vi "VP_RT_MultiTraj.vi"() -> ()   [LabVIEW 2015]
uses:
  Local or Remote.ctl
  State Enum.ctl
  Command Enum.ctl
  Controller Type.ctl
  EPICS Command Control.ctl
  <vilib>/Platform/TimedLoop/XDataNode/timing_clust.ctl
  <vilib>/Platform/TimedLoop/XDataNode/nitl_modes.ctl
  <vilib>/Platform/TimedLoop/XDataNode/wakeup.ctl
  Data Write Control.ctl
  <vilib>/FPGAPlugInAG/cRIO-9039/niLvFpga_Open_cRIO-9039.vi
  <vilib>/rvi/interface/common/dynamic/niFpgaDynamicAddResources.vi
  <vilib>/Utility/error.llb/Error Cluster From Error Code.vi
  <vilib>/rvi/errors/niLvFpgaAdjustHostInterfaceError.vi
  <vilib>/rvi/interface/common/niFpgaWaitOnOcc.vi
  <vilib>/FPGAPlugInAG/Dynamic/niLvFpga_Reset_Dynamic.vi
  <vilib>/FPGAPlugInAG/Dynamic/niLvFpga_Abort_Dynamic.vi
  <vilib>/FPGAPlugInAG/Dynamic/niLvFpga_Close_Dynamic.vi
  <vilib>/Platform/TimedLoop/XDataNode/XDataNode.xnode
  <vilib>/rvi/interface/nirviOpenFPGA/nirviOpenFPGA.xnode
  FPGA Bitfiles/VP_NanoPositioner_FPGA_MultiTraj.lvbitx
  <vilib>/rvi/interface/nirviReadWriteControl/nirviReadWriteControl.xnode
  <vilib>/rvi/interface/nirviMethod/nirviMethod.xnode
  <vilib>/rvi/interface/nirviCloseFPGA/nirviCloseFPGA.xnode
  <vilib>/Platform/TimedLoop/XDataNode/XDNodeRunTimeDep.lvlib
  <vilib>/rvi/errors/niLvFpgaMergeErrorWithErrorCode.vi
  NiFpgaLv.dll
  <vilib>/rvi/interface/Simulation/niFpgaSimulationCallBeginRW.vi
  <vilib>/rvi/Analysis/host/Public/NI_FpgaMspHost.lvlib
  <vilib>/FPGAPlugInAG/Dynamic/niLvFpga_StopFifo_Dynamic.vi
  <vilib>/FPGAPlugInAG/Dynamic/niLvFpga_ReadFifo_Dynamic.vi
  <vilib>/NI_Real-Time Target Support.lvlib
  <vilib>/FPGAPlugInAG/Dynamic/niLvFpga_ConfigureFifo_Dynamic.vi
  <vilib>/FPGAPlugInAG/Dynamic/niLvFpga_StartFifo_Dynamic.vi
panel:
  out "Kzz Output, Kzz*ez (V)":fxp<+/-,58,25>
  out "Kyy Output, Kyy*ey (V)":fxp<+/-,58,25>
  out "Kxx Output, Kxx*ex (V)":fxp<+/-,58,25>
  out "Controller Output Upper Limit Readback":fxp<+/-,20,5>
  out "Controller Output Lower Limit Readback":fxp<+/-,20,5>
  out "X-Stage Input In Range?":bool=TRUE
  out "Y-Stage Input In Range?":bool=TRUE
  out "Z-Stage Input In Range?":bool=TRUE
  in  "Tab Control":T1(tab)
  in  "Controller Type":T2
  in  "X Ramp Start (nm)":fxp<+/-,32,16>=-500.0
  in  "X Ramp End (nm)":fxp<+/-,32,16>=500.0
  in  "Y Ramp Start (nm)":fxp<+/-,32,16>=500.0
  in  "Y Ramp End (nm)":fxp<+/-,32,16>=-500.0
  in  "Y Step Size (nm)":fxp<+/-,32,16>=50.0
  in  "X Step Size (nm)":fxp<+/-,32,16>=50.0
  in  "System Loop Type":enum16{"Open Loop", "Closed Loop"}(ring)
  in  "DT Frequency (Hz)":dbl=1000.0 format="%#_6p"
  in  "DT duty cycle (%)":dbl=88.0 min=0.0 max=100.0 step=1.0
  in  "Max radius":fxp<+/-,32,16>
  in  "Spiral Step Size":fxp<+/-,32,16>
  in  "Scan Geometry":T3(ring)
  in  "Inner Scan axis":enum16{"X", "Y"}(ring)
  in  "Rotation Direction":enum16{"Clockwise", "Anti-clockwise"}(ring)
  in  "Radial direction":enum16{"Outward", "Inward"}(ring)
  out "Trajectory Completed":bool
  out "XY Ref":cluster{dbl[], dbl[]}[](graph)
  out "Elements Available in FIFO":u32(graph)
  out "Elements Remaining in FIFO":u32(graph)
  out "Reference and Actual positions":cluster{"t0":dbl, dbl, dbl[][]}(graph)
  in  "Timeout FPGA FIFO1":i32=40000000
  out "FIFO Timed Out":bool
  out "Stop Run":bool
  in  "Datalog Cases":T4(ring)=enum."Data Log 16"
  out "FIFO Timed Out?":bool
  out "Data Read Rate (Hz)":dbl=25000.000000000004
  out "Elements Remaining":u32
  in  "FIFO Timeout (ms)":i32=2500
  out "Actual Depth":u32=131068416
  in  "Requested Depth":u32=131068000
  in  "Fly scan loop dt":i64=250
  in  "Start Scan Loop dt":i64=50
  out "Queue is empty":bool=TRUE
  out "2iddVELO:VP:X_End_nm":dbl=2000.0
  out "2iddVELO:VP:X_Start_nm":dbl=-2000.0
  out "EPICS Execute Command":bool
  out "2iddVELO:VP:Y_Start_nm":dbl=2000.0
  out "2iddVELO:VP:Y_End_nm":dbl=-2000.0
  out "2iddVELO:VP:Y_Step_Size_nm":dbl=50.0
  out "2iddVELO:VP:X_Step_Size_nm":dbl=50.0
  out "2iddVELO:VP:Trigger_Freq_Hz":dbl=1000.0
  out "2iddVELO:VP:Trig_DutyCycle_Per":dbl=99.0
  out "Remote Mode":bool
  out "EPICS Controller Type":T2
  out "EPICS cRIO Command":T5
  out "EPICS Scan Trajectory":T3(ring)
  out "2iddVELO:VP:Max_Radius":dbl
  out "2iddVELO:VP:Spiral_Step":dbl
  out "Iteration Duration RT Timed-Loop":i64=128
  out "# of Hor Lines":fxp<+/-,64,34>=181.0 format="%.22g"
  out "# of Points per Line":fxp<+/-,33,17>=180.0
  out "# Total Trigger Points":fxp<+/-,64,34>=32580.0
  out "sec per line":dbl=0.06
  out "line per sec (Hz)":dbl=16.666666666666668
  out "Total Scan Time (sec)":dbl=10.86
  in  "Controller Time Period (uSec)":u32=40
  in  "Controller Output Time Period (uSec)":u32=40
  in  "XY Reference Time Period (uSec)":u32=40
  in  "Plant Output Time Period (uSec)":u32=40
  in  "Datalog Time Period (uSec)":u32=40
  in  "Trigger Generation Time Period (uSec)":u32=40
  in  "Z Reference Time Period (uSec)":u32=40
  in  "Stop System (Careful!!)":bool
  in  "Reset All":bool
  in  "Base name":string="base_name"
  out "Mod6/DIO3":bool
  out "Mod5/DIO3":bool
  out "Mod4/DIO3":bool
  in  "Sample Z Stage Resolution (nm)":fxp<+,33,3>=0.5
  in  "Sample Y Stage Resolution (nm)":fxp<+,33,3>=0.5
  in  "Sample X Stage Resolution (nm)":fxp<+,33,3>=0.5
  in  "Optics Z Stage Resolution (nm)":fxp<+,33,3>=0.5
  in  "Optics Y Stage Resolution (nm)":fxp<+,33,3>=0.5
  in  "Optics X Stage Resolution (nm)":fxp<+,33,3>=0.5
  in  "Sample Z Reset":bool
  in  "Sample Y Reset":bool
  in  "Sample X Reset":bool
  out "Mod6/DIO2":bool
  out "Mod6/DIO1":bool
  out "Mod6/DIO0":bool=TRUE
  out "Mod5/DIO2":bool
  out "Mod5/DIO1":bool=TRUE
  out "Mod5/DIO0":bool
  out "Mod4/DIO2":bool=TRUE
  out "Mod4/DIO1":bool
  out "Mod4/DIO0":bool=TRUE
  in  "Optics Z Reset":bool
  in  "Optics Y Reset":bool
  in  "Optics X Reset":bool
  in  "Detector Trigger Lower Limit (V)":fxp<+/-,20,5>
  in  "Detector Trigger Upper Limit (V)":fxp<+/-,20,5>=5.0
  out "Detector Trigger In Range?":bool=TRUE
  in  "DT Reference Amplitude (V)":fxp<+/-,40,17>=5.0
  in  "DT Reference DC Offset (V)":fxp<+/-,16,16>
  out "DT Frequency (periods/tick)":fxp<+,32,0>=7.500010542571545e-05
  out "DT Phase Offset (periods)":fxp<+,32,0>
  in  "DT Reset":bool
  out "DT Duty Cycle (periods)":fxp<+,32,0>=0.8799999998882413
  in  "DT phase offset (deg)":dbl format="%#.6g"
  out "Trigger Frequency (Hz)":dbl
  out "Trigger Duty Cycle (%)":dbl
  in  "Scaling mV to V":fxp<+,33,10>=0.001000046730041504
  out "Heartbeat":bool=TRUE
  in  "System command":T6
  in  "Execute":bool
  out "Last Command Executed":T6
  in  "Optics and or Sample Stage":T7(ring)
  in  "Local_Lock":bool
  out "Local or EPICS":T8
  out "Output filename":string
  out "Output path":path
  out "FPGA state":T9(ring)
  in  "cRIO data dir":string="/home/lvuser/natinst/data"
  out "RT Main Loop State":T10
  out "cRIO path":path
  out "Iteration Duration":i64
  out "Controller loop iterations":i32
  out "Z Reference Loop iterations":i32
  out "XY Reference Loop iterations":i32
  out "FIFO loop iterations":i32
  out "Trigger Generation Loop iterations":i32
  out "Module output loop iterations":i32
  out "Plant output loop iterations":i32
  in  "Data Save Trigger Source":enum16{"Detector", "Trajectory"}(ring)
  out "EPICS rotation direction":enum16{"Clockwise", "Anti-clockwise"}(ring)
  out "EPICS radial direction":enum16{"Outward", "Inward"}(ring)
  out "EPICS Inner axis":enum16{"X", "Y"}(ring)
  out "Optics Z Stage Displacement (nm)":fxp<+/-,32,16>
  out "Optics Y Stage Displacement (nm)":fxp<+/-,32,16>
  out "Optics X Stage Displacement (nm)":fxp<+/-,32,16>=-1.0
  in  "Scan type":enum16{"Fly", "Step"}(ring)
  out "EPICS Scan Type":enum16{"Fly", "Step"}(ring)
  out "Counter Loop iterations":i32
  out "Outer Loop iterations":i32
  out "Scan Type and Geometry":T11(ring)
  out "Position Number":u32
  in  "Data Save Flag":enum16{"Skip Data", "Save Data"}(ring)=enum."Save Data"
  in  "Z-Stage Scaling Direction":fxp<+/-,3,3>=-1.0
  in  "Y-Stage Scaling Direction":fxp<+/-,3,3>=-1.0
  in  "Z-Stage nm to V Scaling":fxp<+/-,32,12>=0.0005397796630859375
  in  "Y-Stage nm to V Scaling":fxp<+/-,32,12>=0.0014200210571289062
  in  "X-Stage Scaling Direction":fxp<+/-,3,3>=-1.0
  in  "X-Stage nm to V Scaling":fxp<+/-,32,12>=0.0005359649658203125
  in  "Controller Output Lower Limit":fxp<+/-,20,5>=-5.0
  in  "Controller Output Upper Limit":fxp<+/-,20,5>=5.0
  in  "FPGA Wait Timer (ms)":u16=5
  in  "Pre-Scan pause (ms)":u32=250
  in  "Readback Loop time between iterations (ms)":u32=10
  in  "Z Reference DC Offset (nm)":fxp<+/-,15,15>
  in  "Y Reference DC Offset (nm)":fxp<+/-,16,16>
  in  "X Reference DC Offset (nm)":fxp<+/-,16,16>
  in  "Z Reference Amplitude (nm)":fxp<+/-,40,17>
  in  "Y Reference Amplitude (nm)":fxp<+/-,40,17>=100.0
  in  "X Reference Amplitude (nm)":fxp<+/-,40,17>=100.0
  out "Trajectory frequency (periods/tick)":fxp<+,32,0>=1.25030055642128e-07 format="%#.5e"
  in  "Trajectory frequency (Hz)":dbl=25000.0 format="%#_6p"
  out "actual Traj frequency (Hz)":dbl format="%#_6p"
  out "Measured Datalog Time Period (Ticks)":u32=1600
  out "Measured Datalog Loop Rate (us)":dbl=3.9999999999999996e-05
  out "Measured Datalog Loop Rate (kHz)":dbl=25.000000000000004
  out "Measured Counter Loop Rate (us)":dbl
  out "Measured Counter Loop Rate (MHz)":dbl=inf
  out "Measured XY Reference Loop Rate (us)":dbl=3.9999999999999996e-05
  out "Measured XY Reference Loop Rate (kHz)":dbl=25.000000000000004
  out "Measured XY Reference Time Period (Ticks)":u32=1600
  out "Measured Controller Loop Rate (kHz)":dbl=25.000000000000004
  out "Measured Controller Output Loop Rate (us)":dbl=3.9999999999999996e-05
  out "Measured Controller Output Loop Rate (kHz)":dbl=25.000000000000004
  out "Measured Plant Output Loop Rate (us)":dbl=3.9999999999999996e-05
  out "Measured Plant Output Loop Rate (kHz)":dbl=25.000000000000004
  out "Measured Controller Loop Rate (us)":dbl=3.9999999999999996e-05
  out "Measured Controller Time Period (Ticks)":u32=1600
  out "Data Read Period (sec)":dbl=3.9999999999999996e-05
  out "Measured Controller Output Time Period (Ticks)":u32=1600
  out "Measured Plant Output Time Period (Ticks)":u32=1600
  out "Measured Counter Time Period (Ticks)":u32
  out "Measured Trigger Gen Time Period (Ticks)":u32=1600
  out "Measured Z Reference Time Period (Ticks)":u32=1600
  out "Measured Z Reference Loop Rate (us)":dbl=3.9999999999999996e-05
  out "Measured Z Reference Loop Rate (kHz)":dbl=25.000000000000004
  out "Number of Data Strings":i32=5
  out "Data":fxp<+/-,40,32>[](array[numeric])
  out "Measured Trigger Gen Loop Rate (us)":dbl=3.9999999999999996e-05
  out "Measured Trigger Gen Loop Rate (kHz)":dbl=25.000000000000004
  in  "file path soscoeff_xx1 Hinf":path=path "/home/lvuser/natinst/controllers/Kxx_1_Gxx_matched_dow_16ord_mVpnm_cd8a3_AvTio9_X5nm_500pm_all_40us_soscof_xx1.mat"
  in  "file path sos gain SF Controller_xx1 Hinf":path=path "/home/lvuser/natinst/controllers/Kxx_1_Gxx_matched_dow_16ord_mVpnm_cd8a3_AvTio9_X5nm_500pm_all_40us_soscof_xx2.mat"
  in  "file path soscoeff_yy1 Hinf":path=path "/home/lvuser/natinst/controllers/Kyy_trial_1_Gyy_matched_dow_8ord_mVpnm_cd8a3_AvTio9_Y5nm_500pm_all_40us_soscof_yy1.mat"
  in  "file path sos gain SF Controller_yy1 Hinf":path=path "/home/lvuser/natinst/controllers/Kyy_trial_1_Gyy_matched_dow_8ord_mVpnm_cd8a3_AvTio9_Y5nm_500pm_all_40us_soscof_yy2.mat"
  in  "file path soscoeff_zz1 Hinf":path=path "/home/lvuser/natinst/controllers/Kzz_1_Gzz_matched_dow_29ord_mVpnm_cd8a3_AvTio9_Z5nm_500pm_all_40us_soscof_zz1.mat"
  in  "file path sos gain SF Controller_zz1 Hinf":path=path "/home/lvuser/natinst/controllers/Kzz_1_Gzz_matched_dow_29ord_mVpnm_cd8a3_AvTio9_Z5nm_500pm_all_40us_soscof_zz2.mat"
  in  "file path soscoeff_xx1 PID":path=path "/home/lvuser/natinst/controllers/Kxx_pid_2_Gxx_tustin_2ord_mVpnm_cd8a3_soscof_xx1.mat"
  in  "file path sos gain SF Controller_xx1 PID":path=path "/home/lvuser/natinst/controllers/Kxx_pid_2_Gxx_tustin_2ord_mVpnm_cd8a3_soscof_xx2.mat"
  in  "file path soscoeff_yy1 PID":path=path "/home/lvuser/natinst/controllers/Kyy_pid_4_Gyy_tustin_2ord_mVpnm_cd8a3_soscof_yy1.mat"
  in  "file path sos gain SF Controller_yy1 PID":path=path "/home/lvuser/natinst/controllers/Kyy_pid_4_Gyy_tustin_2ord_mVpnm_cd8a3_soscof_yy2.mat"
  in  "file path soscoeff_zz1 PID":path=path "/home/lvuser/natinst/controllers/Kzz_pid_2_Gzz_tustin_2ord_mVpnm_cd8a3_soscof_zz1.mat"
  in  "file path sos gain SF Controller_zz1 PID":path=path "/home/lvuser/natinst/controllers/Kzz_pid_2_Gzz_tustin_2ord_mVpnm_cd8a3_soscof_zz2.mat"
  out "-a01(2) xx1c":fxp<+/-,64,9>[](array[numeric])=[0.637785025840232, 0.9924182654286198, 1.8461027816316544, 0.8635404845716299, 1.0670555456779864, 1.6350703383821101, 1.6323955588345012, 1.1102241390539636, 0.0, 0.0, 0.0, 0.0, 0.0, 0.0, 0.0, 0.0, 0.0, 0.0, 0.0, 0.0]
  out "-a02(2) xx1c":fxp<+/-,64,9>[](array[numeric])=[-0.999855815746439, -0.9676991072632725, -0.9642268720534838, -0.9446498323360957, -0.9442808087139987, -0.7547983908829242, -0.6690016013017409, -0.11027986125857198, 0.0, 0.0, 0.0, 0.0, 0.0, 0.0, 0.0, 0.0, 0.0, 0.0, 0.0, 0.0]
  out "b01(2) xx1c":fxp<+/-,64,9>[](array[numeric])=[-0.6378105164532328, -1.0062332697665268, -1.8762916543815855, -0.8616288879491845, -1.0856571140792324, -1.6862585929720944, -1.743591709663851, -0.6129835805090948, 0.0, 0.0, 0.0, 0.0, 0.0, 0.0, 0.0, 0.0, 0.0, 0.0, 0.0, 0.0]
  out "b02(2) xx1c":fxp<+/-,64,9>[](array[numeric])=[0.9999102047610771, 0.9971375605901365, 0.9926840301018772, 0.9509648854364836, 0.9563369558920378, 0.7818900462139817, 0.7642575436257291, 3.0531133177191805e-16, 0.0, 0.0, 0.0, 0.0, 0.0, 0.0, 0.0, 0.0, 0.0, 0.0, 0.0, 0.0]
  out "sos gain SF Controller xx1c":fxp<+/-,42,9>=-0.1625035791657865
  out "-a01(2) yy1c":fxp<+/-,64,9>[](array[numeric])=[1.8740229377643998, 1.3096977339382483, 1.7453886241944765, 0.2668895009727739, 0.0, 0.0, 0.0, 0.0, 0.0, 0.0, 0.0, 0.0, 0.0, 0.0, 0.0, 0.0, 0.0, 0.0, 0.0, 0.0]
  out "-a02(2) yy1c":fxp<+/-,64,9>[](array[numeric])=[-0.9732703278433918, -0.5194903821190732, -0.7453924481836136, -2.7755575615628914e-17, 0.0, 0.0, 0.0, 0.0, 0.0, 0.0, 0.0, 0.0, 0.0, 0.0, 0.0, 0.0, 0.0, 0.0, 0.0, 0.0]
  out "b01(2) yy1c":fxp<+/-,64,9>[](array[numeric])=[-1.8979173162254057, -1.8463149313261074, -1.7151162246453355, -0.006444279582847878, 0.0, 0.0, 0.0, 0.0, 0.0, 0.0, 0.0, 0.0, 0.0, 0.0, 0.0, 0.0, 0.0, 0.0, 0.0, 0.0]
  out "b02(2) yy1c":fxp<+/-,64,9>[](array[numeric])=[0.9969084979865663, 0.9421233904433339, 0.7362048104846675, 0.0, 0.0, 0.0, 0.0, 0.0, 0.0, 0.0, 0.0, 0.0, 0.0, 0.0, 0.0, 0.0, 0.0, 0.0, 0.0, 0.0]
  out "sos gain SF Controller yy1c":fxp<+/-,42,9>=-1.480983349494636
  out "-a01(2) zz1c":fxp<+/-,64,9>[](array[numeric])=[0.6242394224317618, 1.8967038692417004, 0.6659160318030806, 1.7792660019034106, 1.6870099721477447, 0.6417945190222861, 1.4838029149808185, 1.8456549628851837, 1.2189509782386598, 0.9933314517253298, 1.0158915520299678, 0.8863484387433826, 0.026837806879254994, 1.8269783715122585, 0.22448441435364225, 0.0, 0.0, 0.0, 0.0, 0.0]
  out "-a02(2) zz1c":fxp<+/-,64,9>[](array[numeric])=[-0.9983298461163967, -0.9972287452752734, -0.995744457243837, -0.9947210838396919, -0.9925914602095722, -0.9920974045271405, -0.9881915357970101, -0.9800069383591395, -0.9760641145386646, -0.9508624135515895, -0.9242774595356998, -0.655945641403593, -0.008661844724279444, -0.8269827070369743, 0.0, 0.0, 0.0, 0.0, 0.0, 0.0]
  out "b01(2) zz1c":fxp<+/-,64,9>[](array[numeric])=[-0.6245671059510156, -1.897930093390194, -0.6670970070931089, -1.7670265604573054, -1.6833314913922348, -0.6327437892303018, -1.5025901530730128, -1.8636454269915796, -1.1210694827766767, -0.9982206064398196, -1.0326369335418408, -1.1342635673267367, -1.6852506306166828, -0.9843740162364313, -1.7208456881689926e-15, 0.0, 0.0, 0.0, 0.0, 0.0]
  out "b02(2) zz1c":fxp<+/-,64,9>[](array[numeric])=[0.9973135069419645, 0.9951302056171929, 0.9993435624612031, 0.9919371251860779, 0.994931751453586, 0.9881092761723503, 0.9884874399279107, 0.9977145546300196, 0.9725302934743221, 0.9855561672767964, 0.9893454712398023, 0.846212786518208, 0.7855598927779743, 0.0978075435519738, 0.0, 0.0, 0.0, 0.0, 0.0, 0.0]
  out "sos gain SF Controller zz1c":fxp<+/-,42,9>=-0.1988595259608701
  out "FPGA error monitor":errorcluster
  out "FPGA end run error":errorcluster
  out "Timed Loop (end error)":errorcluster
  out "Main Loop error":errorcluster
  out "Main Loop Iterations":i32
  out "RT error":errorcluster
  out "Command Loop Error":errorcluster
  out "Readback error":errorcluster
  out "FPGA wait error":errorcluster
  out "Coeff file import error":errorcluster
  out "Readback loop Iterations":i32
  out "Command Loop Iterations":i32
  out "Heartbeat Loop Iterations":i32
  out "EPICS command error":errorcluster
  out "FPGA Run Loop error":errorcluster
  out "File Writer loop error":errorcluster
  out "File writer loop iterations":i32
  out "Reduced Array of States":T10[](array[typedef])
  out "2iddVELO:VP:Scan_Type":string
  out "2iddVELO:VP:Controller_Type":string
  out "2iddVELO:VP:cRIO_Command":string
  out "2iddVELO:VP:Scan_Trajectory":string
  out "2iddVELO:VP:Radial_Direction":string
  out "2iddVELO:VP:Rotation_Direction":string
  out "2iddVELO:VP:Inner_Scan_Axis":string
  out "2iddVELO:VP:X_Center":dbl
  out "2iddVELO:VP:Y_Center":dbl
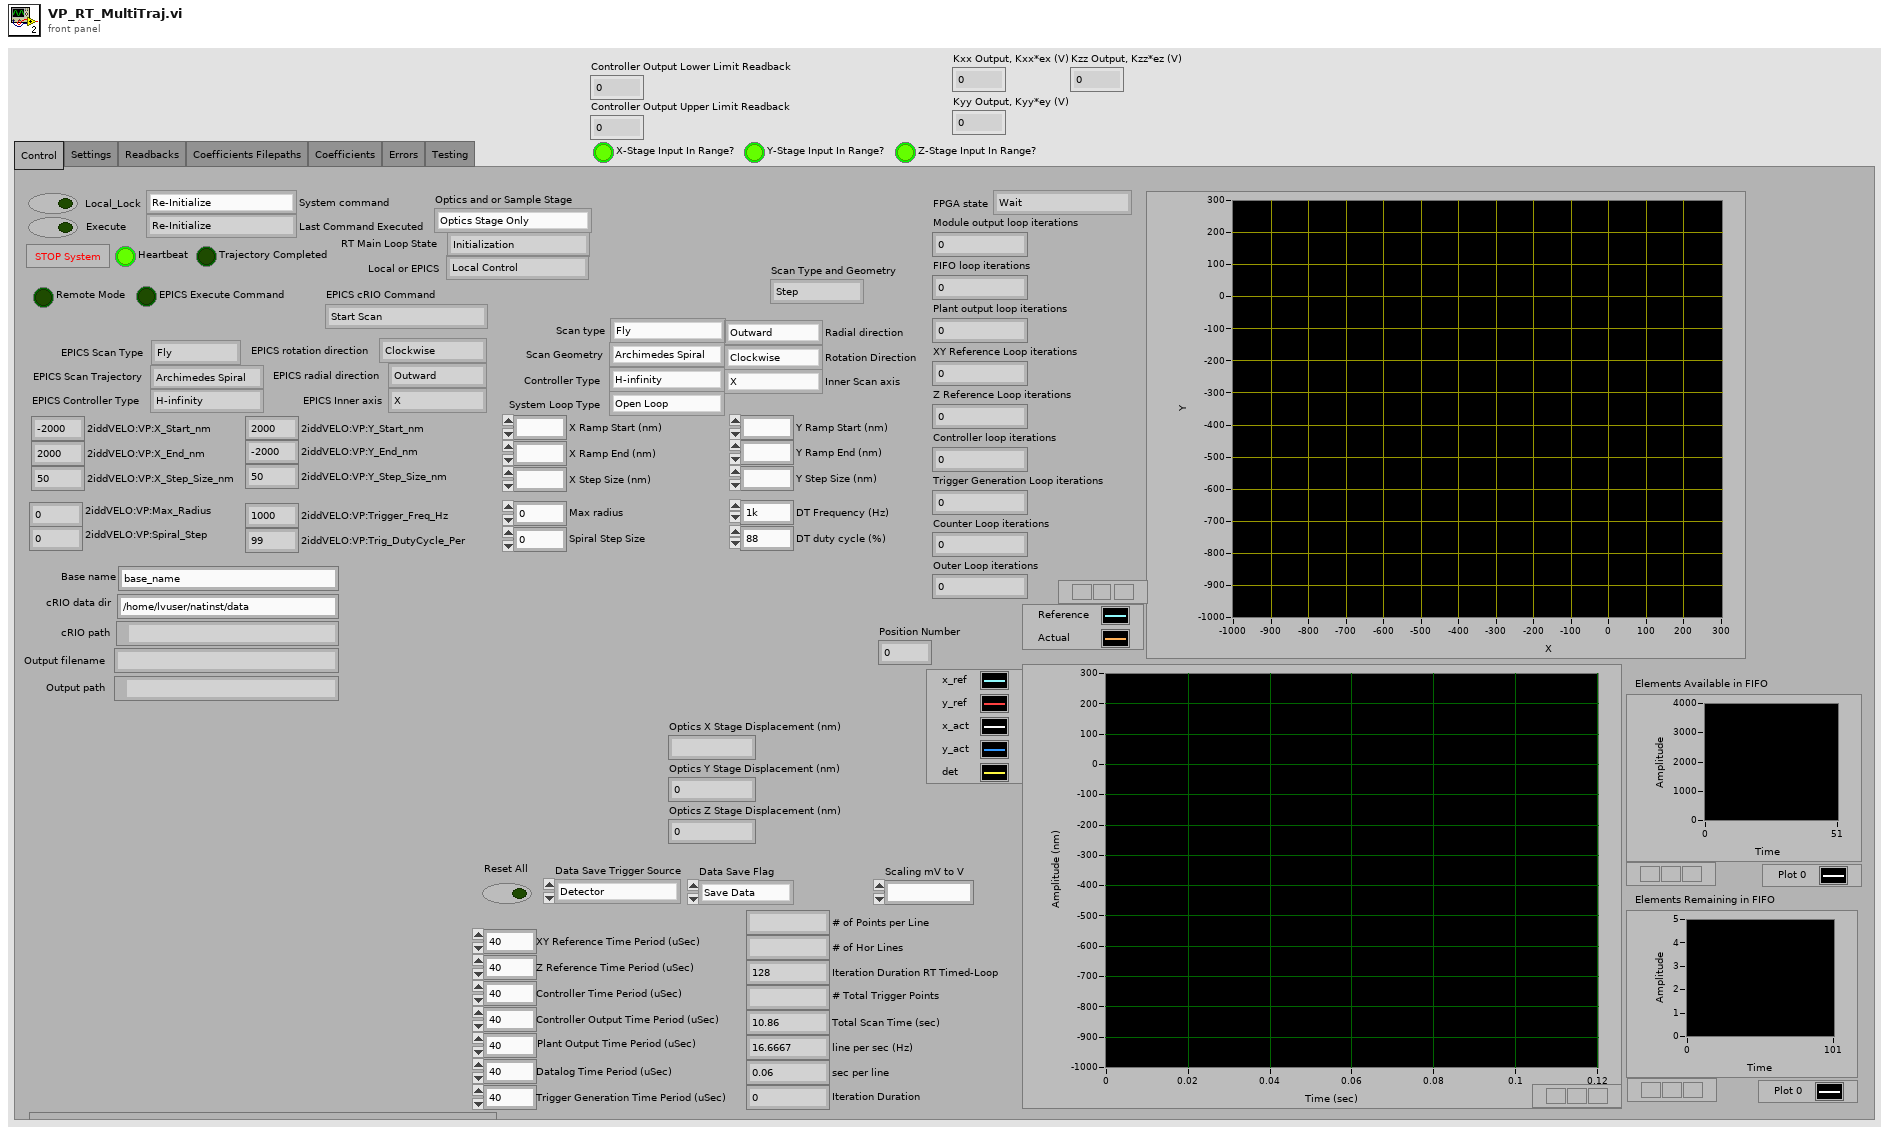
[diagram p1: front panel]
types:
  T1 = enum32{"Control", "Settings", "Readbacks", "Coefficients Filepaths", "Coefficients", "Errors", "Testing"}
  T2 = typedef "Controller Type.ctl" = enum16{"H-infinity", "PID"}
  T3 = enum16{"Archimedes Spiral", "Grid Spiral", "Snake"}
  T4 = enum16{"Data Log 1", "Data Log 2", "Data Log 3", "Data Log 4", "Data Log 5", "Data Log 6", "Data Log 7", "Data Log 8", "Data Log 9", "Data Log 10", "Data Log 11", "Data Log 12", "Data Log 13", "Data Log 14", "Data Log 15", "Data Log 16"}
  T5 = typedef "EPICS Command Control.ctl" = enum16{"Start Scan", "Stop Scan", "Reload Controller"}
  T6 = typedef "Command Enum.ctl" = enum16{"Re-Initialize ", "Update Scan Settings", "Scan", "Stop Scan", "Restart FPGA", "Stop System"}
  T7 = enum16{"Optics Stage Only", "Optics and Sample Stage"}
  T8 = typedef "Local or Remote.ctl" = enum16{"Local Control", "EPICS Control"}
  T9 = enum16{"Wait", "Start Run", "Run", "End Run", "Shutdown"}
  T10 = typedef "State Enum.ctl" = enum16{"Initialization", "Import Controller coeffs", "Update Controller Info", "Wait", "Update Reference Info", "Update Detector Trigger Info", "Update Datalog Info", "Check FPGA Status", "Initialize FIFO", "Pre-Scan", "Start Scan", "Step Scanning", "Fly Scanning", "End Scan", "Close File", "Restart FPGA", "Stop FPGA"}
  T11 = enum16{"Step", "Fly Arch Spiral", "Fly Snake", "Fly Grid Spiral"}
  T12 = typedef "XDNodeRunTimeDep.lvlib/timing_clust.ctl" = cluster{"Expected End [f-1]":u64, "Actual End [f-1]":u64, "Finished Late? [f-1]":bool, "Expected End [i-1]":u64, "Actual End [i-1]":u64, "Finished Late? [i-1]":bool, "Expected Start [i]":u64, "Actual Start [i]":u64, "Expected Start [f]":u64, "Actual Start [f]":u64, "Source Name":string, "Structure Name":string, "Period":i64, "Deadline":i64, "Offset":i64, "Start":i64, "Priority":i32, "Timeout":i32, "Mode":T13, "Wakeup Reason":T14, "Error":errorcluster, "Source Type":string, "Secondary Source Type":string, "Global End Time":u64, "Global Start Time":u64, "Frame Duration":u64, "Iteration Duration":u64, "Assigned CPU":i32, "I/O Scan Engine Mode":u32}
  T13 = typedef "XDNodeRunTimeDep.lvlib/nitl_modes.ctl" = enum32{"No Change", "Process missed periods, maintain original phase", "Discard missed periods, maintain original phase", "Process missed periods, ignore original phase", "Discard missed periods, ignore original phase"}
  T14 = typedef "XDNodeRunTimeDep.lvlib/wakeup.ctl" = enum32{"Normal", "Aborted", "Asynchronous wakeup", "Timing source error", "Timed loop error", "Timeout"}
  T15 = typedef "Data Write Control.ctl" = enum16{"Initialize", "Read", "Write", "Close"}
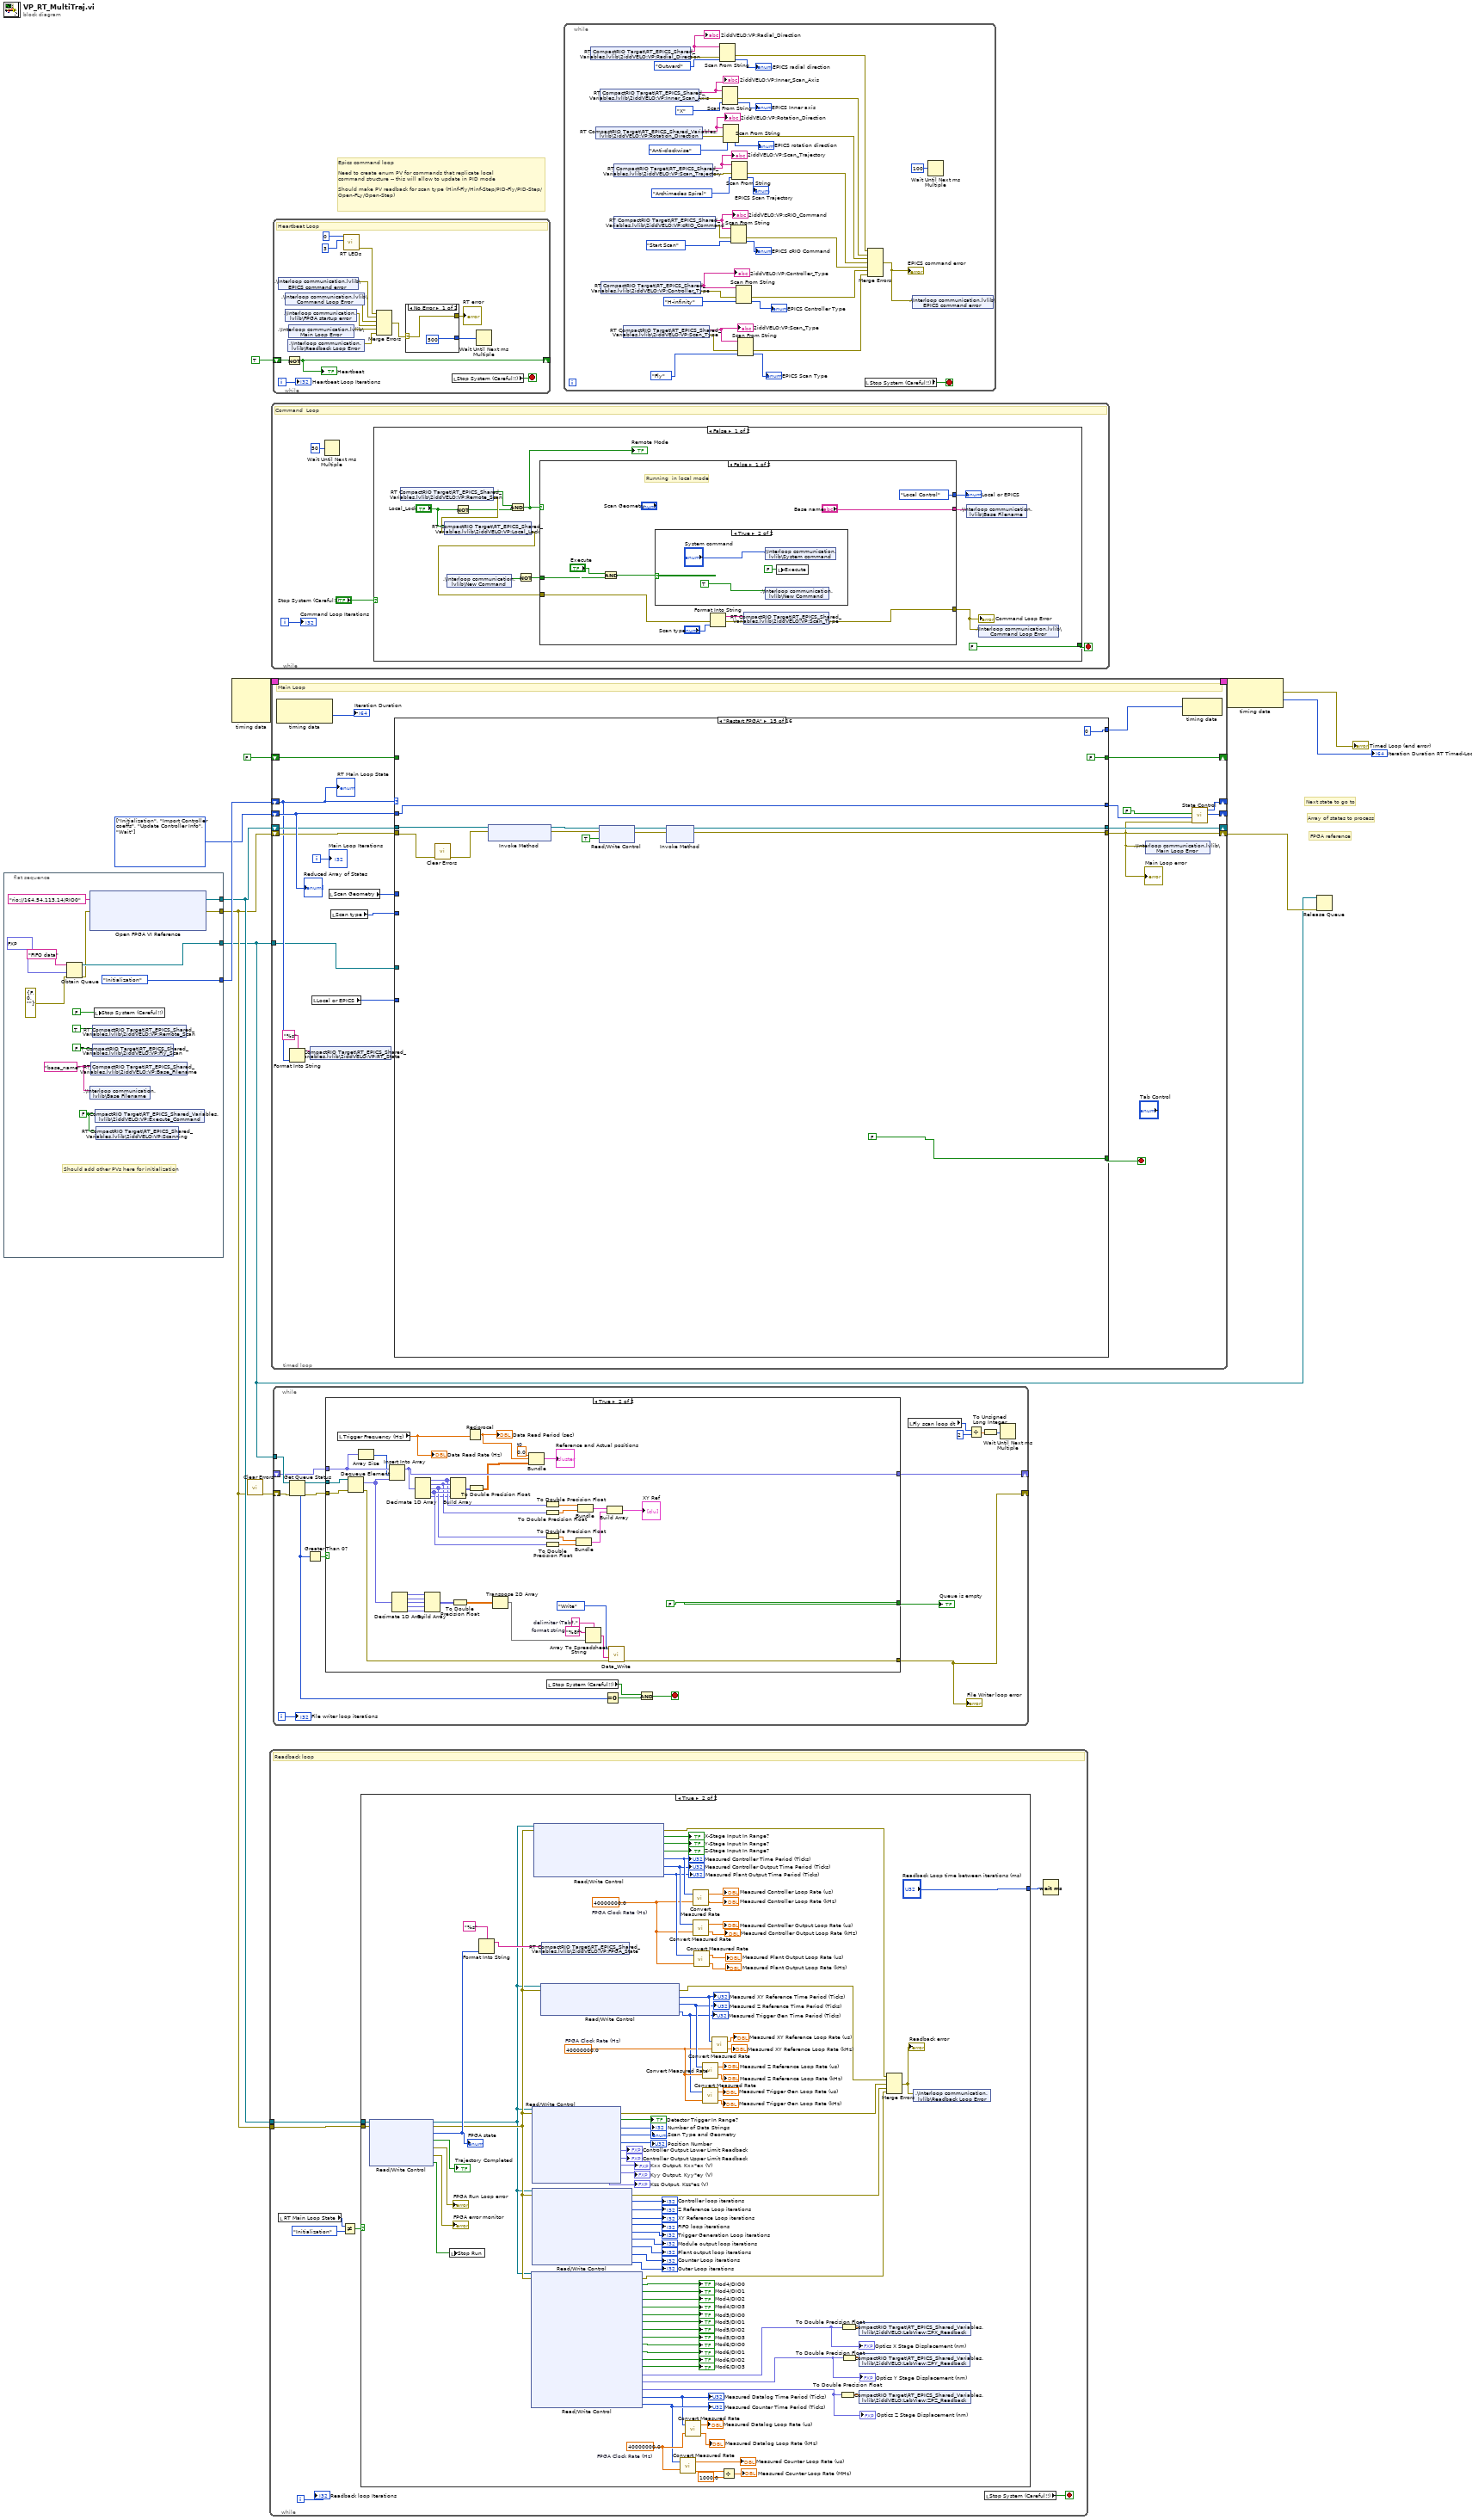
[diagram p0: block diagram]
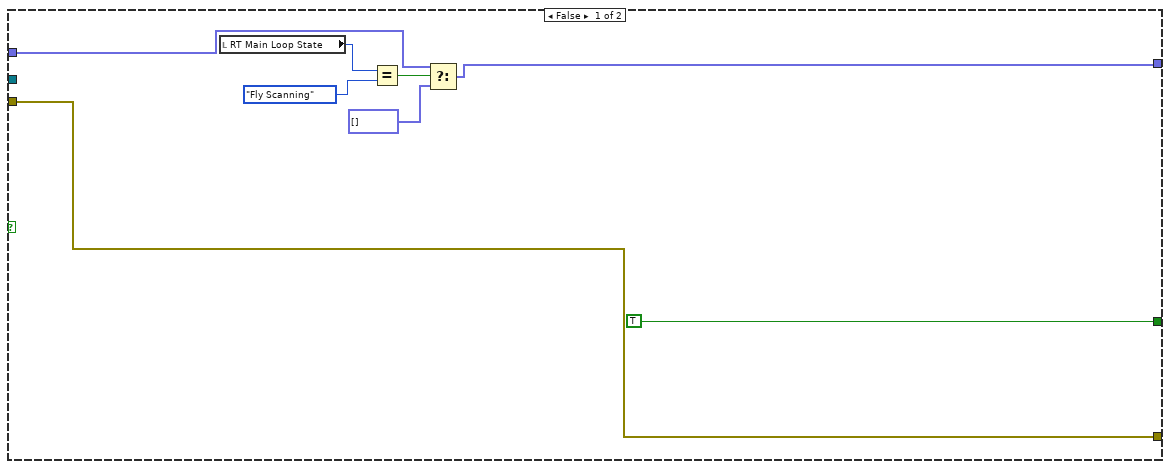
[diagram p2: hidden frame]
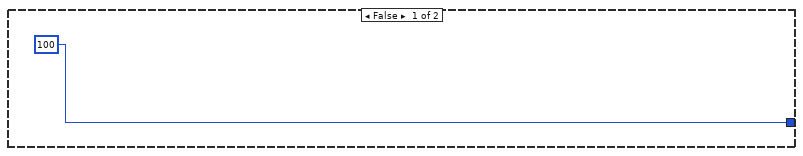
[diagram p3: hidden frame]
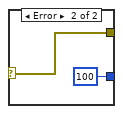
[diagram p4: hidden frame]
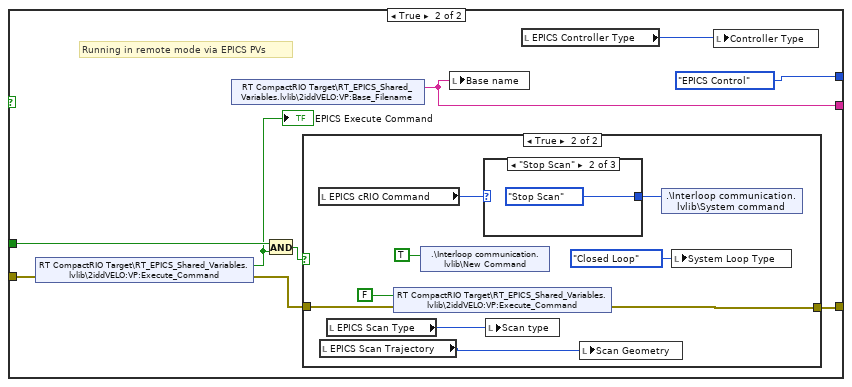
[diagram p6: hidden frame]
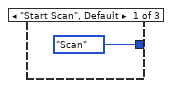
[diagram p8: hidden frame]
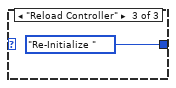
[diagram p9: hidden frame]
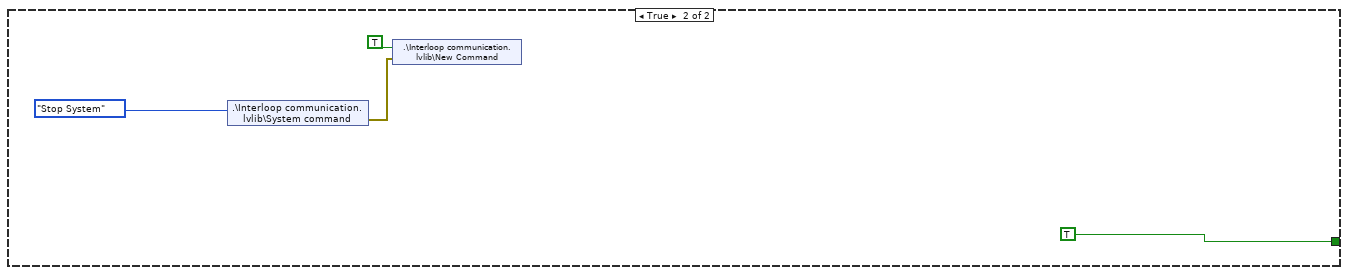
[diagram p10: hidden frame]
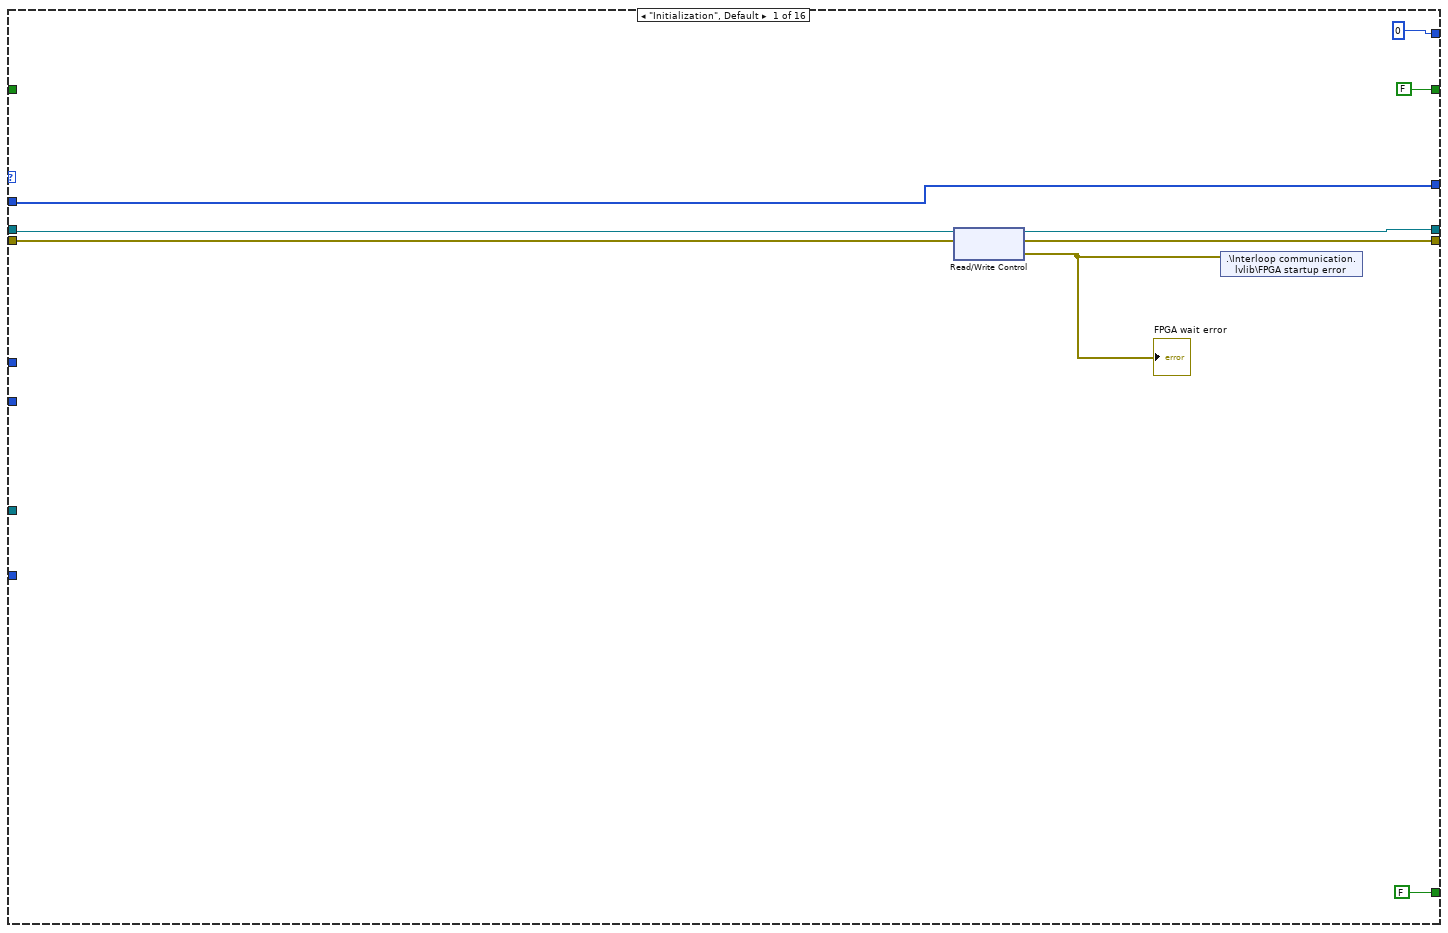
[diagram p11: hidden frame]
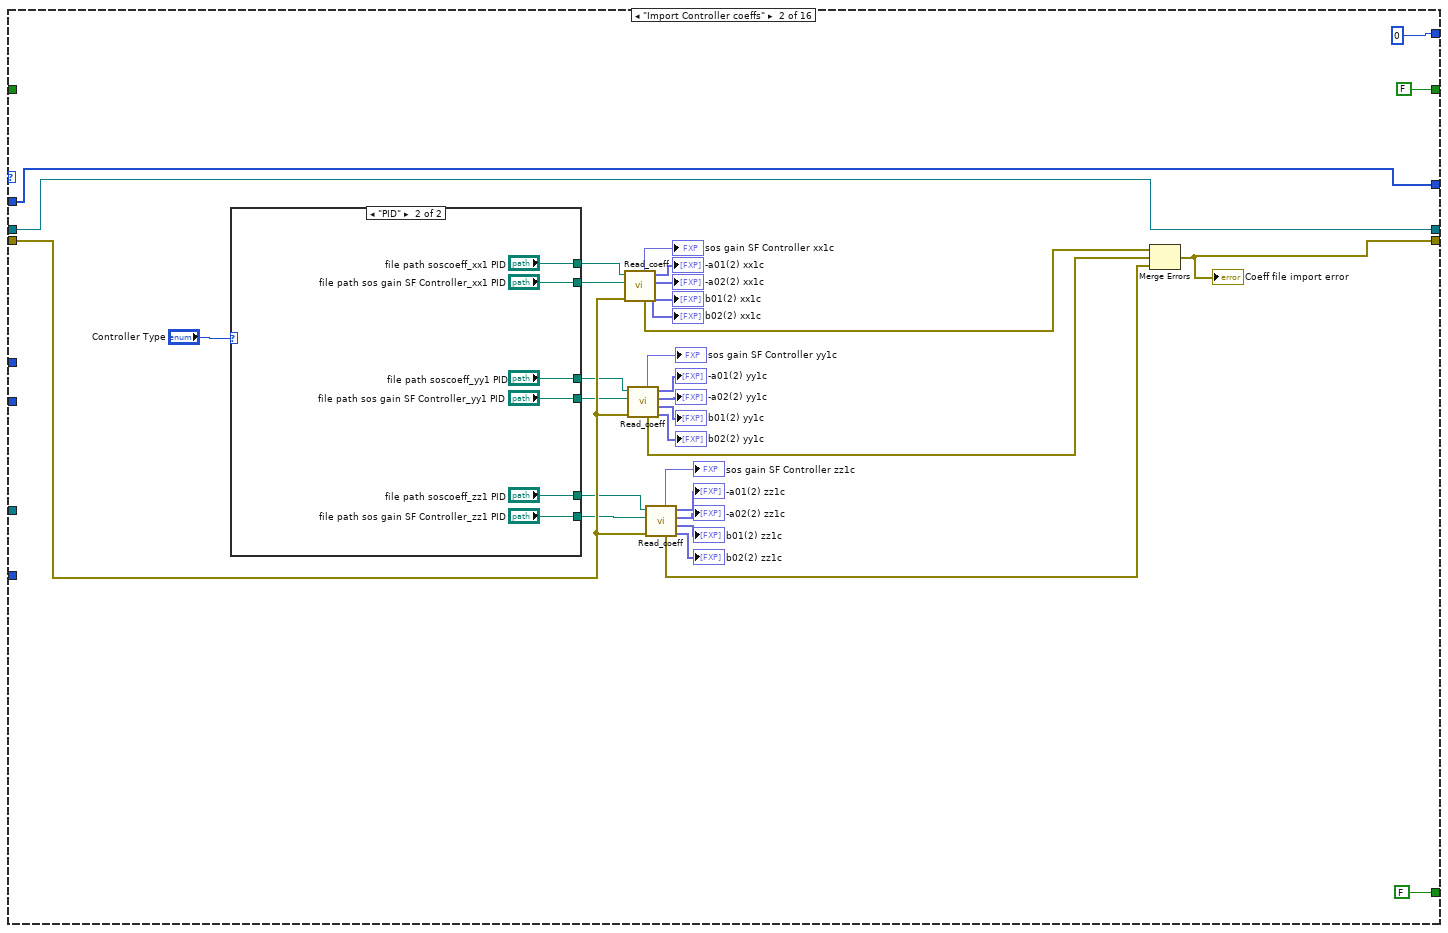
[diagram p12: hidden frame]
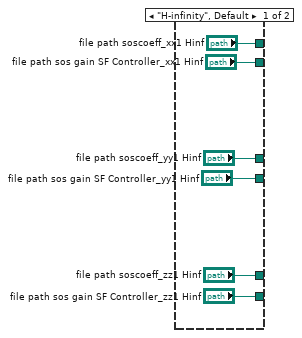
[diagram p13: hidden frame]
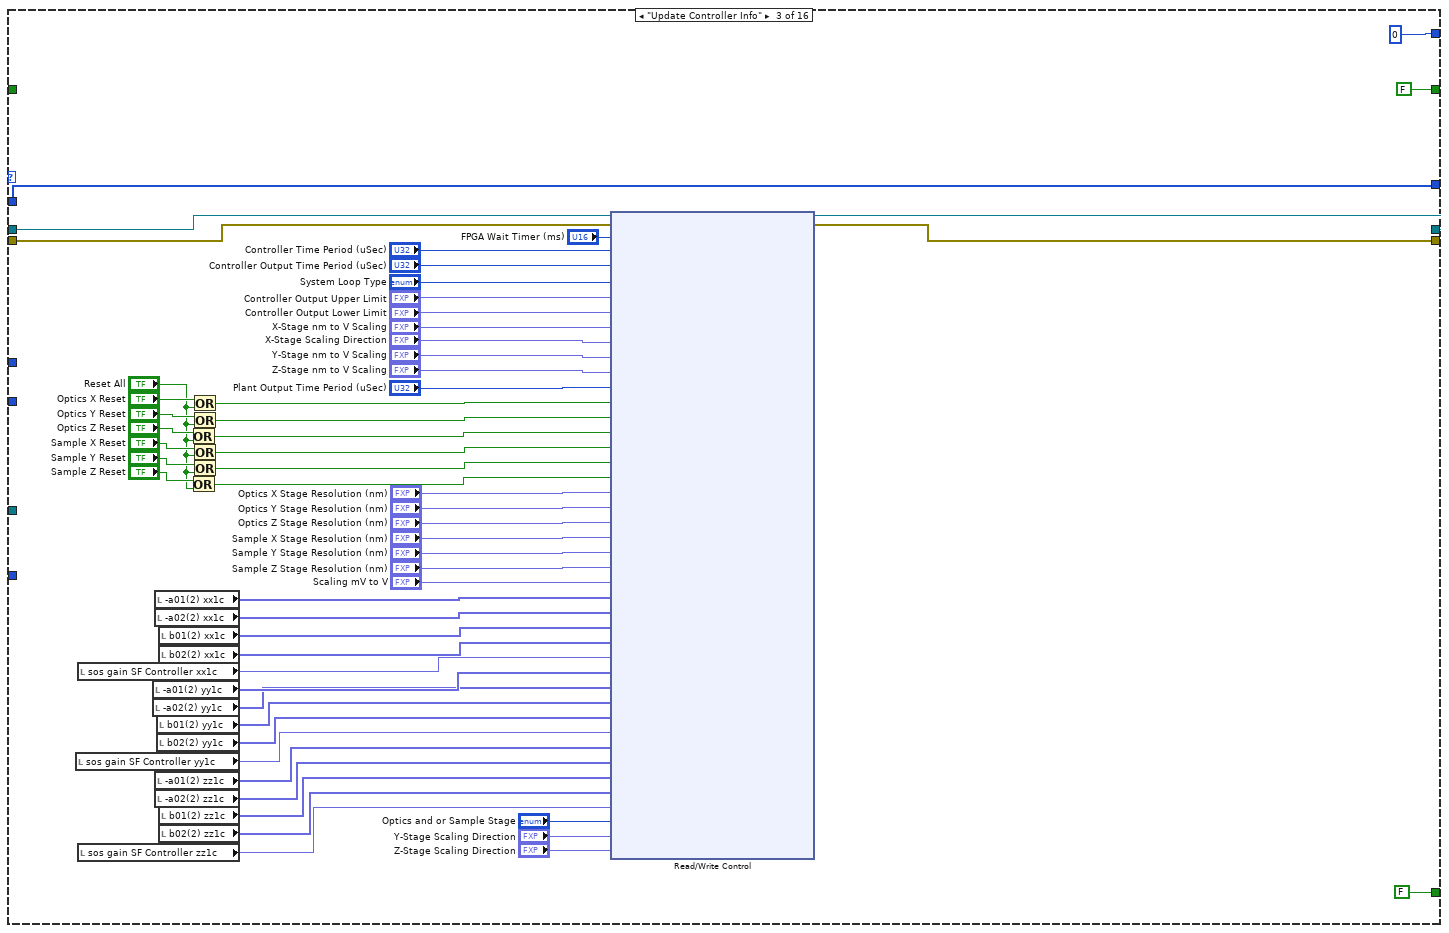
[diagram p14: hidden frame]
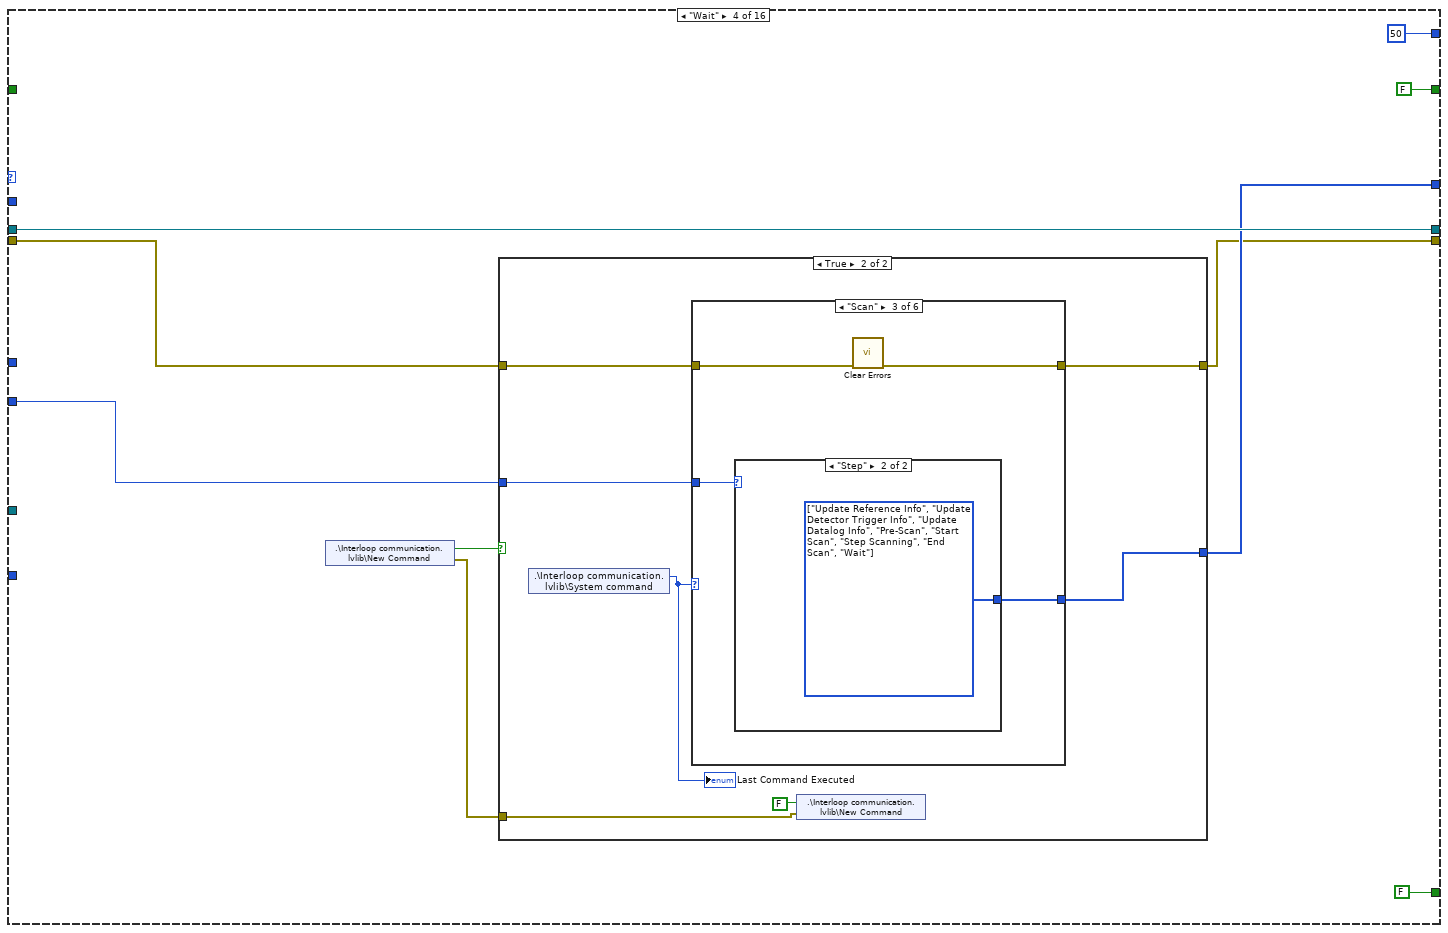
[diagram p15: hidden frame]
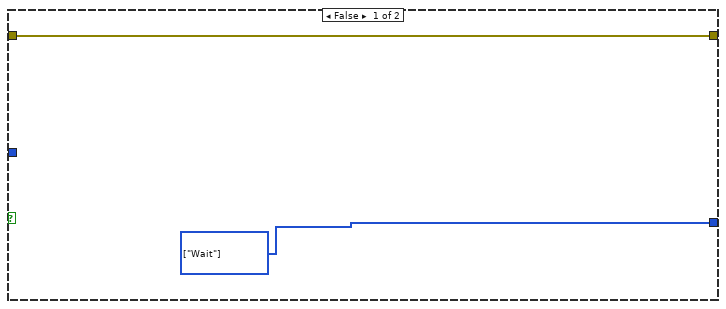
[diagram p16: hidden frame]
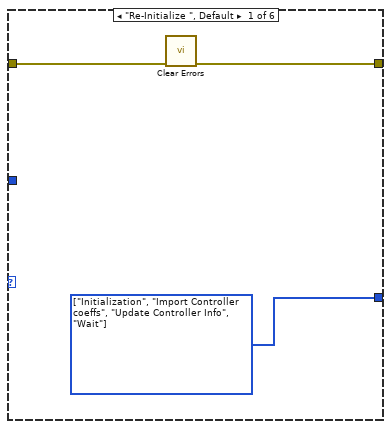
[diagram p17: hidden frame]
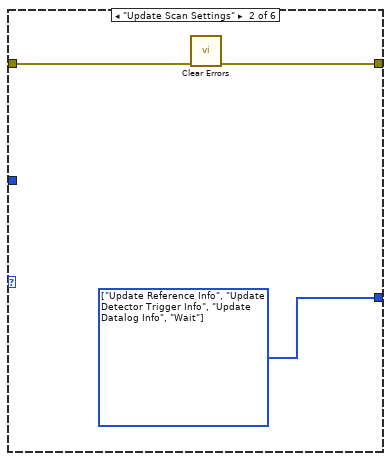
[diagram p18: hidden frame]
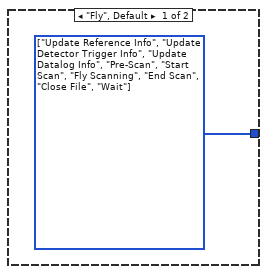
[diagram p19: hidden frame]
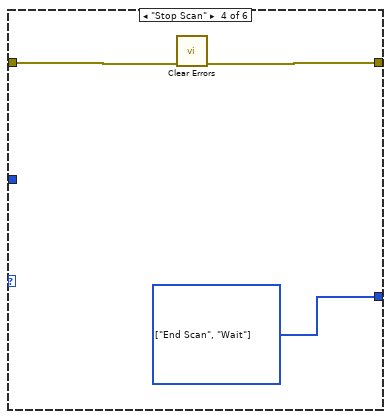
[diagram p20: hidden frame]
diagram:
  w7 = T10[] [enum."Initialization", enum."Import Controller coeffs", enum."Update Controller Info", enum."Wait"] items=["Initialization", "Import Controller coeffs", "Update Controller Info", "Wait", "Update Reference Info", "Update Detector Trigger Info", "Update Datalog Info", "Check FPGA Status", "Initialize FIFO", "Pre-Scan", "Start Scan", "Step Scanning", "Fly Scanning", "End Scan", "Close File", "Restart FPGA", "Stop FPGA"] ("Reduced Array of States")
  # "Epics command loop\n\nNeed to create enum PV for commands that replicate local\ncommand structure -- this will allow to update in PID mode\n\nShould make PV readback for scan type (Hinf-Fly/Hinf-Step/PID-Fly/PID-Step/\nOpen-FLy/Open-Step)"
  # "FPGA reference"
  # "Array of states to process"
  # "Next state to go to"
  n1 = flat-sequence {
    tunnel: [State_Enum."Initialization" ("States")] -> w8
    tunnel: [w25] -> w5
    tunnel: [w24] -> w6
    tunnel: [w17] -> w3
    frame #0 {
      w19 = FALSE ("Start_Scan")
      w22 = "base_name" ("Base_Filename")
      # "Should add other PVs here for initialization"
      n2 = Obtain Queue(name (unnamed)="FIFO data", element data type=fxp<+/-,58,25>[] [0.0, 0.0, 0.0, 0.0, 0.0, 0.0, 0.0, 0.0, 0.0, 0.0, 0.0, 0.0, 0.0, 0.0, 0.0, 0.0, 0.0, 0.0, 0.0, 0.0, 0.0, 0.0, 0.0, 0.0, 0.0, 0.0, 0.0, 0.0, 0.0, 0.0, 0.0, 0.0, 0.0, 0.0, 0.0, 0.0, 0.0, 0.0, 0.0, 0.0, 0.0, 0.0, 0.0, 0.0, 0.0, 0.0, 0.0, 0.0, 0.0, 0.0, 0.0, 0.0, 0.0, 0.0, 0.0, 0.0, 0.0, 0.0, 0.0, 0.0, 0.0, 0.0, 0.0, 0.0, 0.0, 0.0, 0.0, 0.0, 0.0, 0.0, 0.0, 0.0, 0.0, 0.0, 0.0, 0.0, 0.0, 0.0, 0.0, 0.0, 0.0, 0.0, 0.0, 0.0, 0.0, 0.0, 0.0, 0.0, 0.0, 0.0, 0.0, 0.0, 0.0, 0.0, 0.0, 0.0, 0.0, 0.0, 0.0, 0.0, 0.0, 0.0, 0.0, 0.0, 0.0, 0.0, 0.0, 0.0, 0.0, 0.0, 0.0, 0.0, 0.0, 0.0, 0.0, 0.0, 0.0, 0.0, 0.0, 0.0, 0.0, 0.0, 0.0, 0.0, 0.0, 0.0, 0.0, 0.0, 0.0, 0.0, 0.0, 0.0, 0.0, 0.0, 0.0, 0.0, 0.0, 0.0, 0.0, 0.0, 0.0, 0.0, 0.0, 0.0, 0.0, 0.0, 0.0, 0.0, 0.0, 0.0, 0.0, 0.0, 0.0, 0.0, 0.0, 0.0, 0.0, 0.0, 0.0, 0.0, 0.0, 0.0, 0.0, 0.0, 0.0, 0.0, 0.0, 0.0, 0.0, 0.0, 0.0, 0.0, 0.0, 0.0, 0.0, 0.0, 0.0, 0.0, 0.0, 0.0, 0.0, 0.0, 0.0, 0.0, 0.0, 0.0, 0.0, 0.0, 0.0, 0.0, 0.0, 0.0, 0.0, 0.0, 0.0, 0.0, 0.0, 0.0, 0.0, 0.0, 0.0, 0.0, 0.0, 0.0, 0.0, 0.0, 0.0, 0.0, 0.0, 0.0, 0.0, 0.0, 0.0, 0.0, 0.0, 0.0, 0.0, 0.0, 0.0, 0.0, 0.0, 0.0, 0.0, 0.0, 0.0, 0.0, 0.0, 0.0, 0.0, 0.0, 0.0, 0.0, 0.0, 0.0, 0.0, 0.0, 0.0, 0.0, 0.0, 0.0, 0.0, 0.0, 0.0, 0.0, 0.0, 0.0, 0.0, 0.0, 0.0, 0.0, 0.0, 0.0, 0.0, 0.0, 0.0, 0.0, 0.0, 0.0, 0.0, 0.0, 0.0, 0.0, 0.0, 0.0, 0.0, 0.0, 0.0, 0.0, 0.0, 0.0, 0.0, 0.0, 0.0, 0.0, 0.0, 0.0, 0.0, 0.0, 0.0, 0.0, 0.0, 0.0, 0.0, 0.0, 0.0, 0.0, 0.0, 0.0, 0.0, 0.0, 0.0, 0.0, 0.0, 0.0, 0.0, 0.0, 0.0, 0.0, 0.0, 0.0, 0.0, 0.0, 0.0, 0.0, 0.0, 0.0, 0.0, 0.0, 0.0, 0.0, 0.0, 0.0, 0.0, 0.0, 0.0, 0.0, 0.0, 0.0, 0.0, 0.0, 0.0, 0.0, 0.0, 0.0, 0.0, 0.0, 0.0, 0.0, 0.0, 0.0, 0.0, 0.0, 0.0, 0.0, 0.0, 0.0, 0.0, 0.0, 0.0, 0.0, 0.0, 0.0, 0.0, 0.0, 0.0, 0.0, 0.0, 0.0, 0.0, 0.0, 0.0, 0.0, 0.0, 0.0, 0.0, 0.0, 0.0, 0.0, 0.0, 0.0, 0.0, 0.0, 0.0, 0.0, 0.0, 0.0, 0.0, 0.0, 0.0, 0.0, 0.0, 0.0, 0.0, 0.0, 0.0, 0.0, 0.0, 0.0, 0.0, 0.0, 0.0, 0.0, 0.0, 0.0, 0.0, 0.0, 0.0, 0.0, 0.0, 0.0, 0.0, 0.0, 0.0, 0.0, 0.0, 0.0, 0.0, 0.0, 0.0, 0.0, 0.0, 0.0, 0.0, 0.0, 0.0, 0.0, 0.0, 0.0, 0.0, 0.0, 0.0, 0.0, 0.0, 0.0, 0.0, 0.0, 0.0, 0.0, 0.0, 0.0, 0.0, 0.0, 0.0, 0.0, 0.0, 0.0, 0.0, 0.0, 0.0, 0.0, 0.0, 0.0, 0.0, 0.0, 0.0, 0.0, 0.0, 0.0, 0.0, 0.0, 0.0, 0.0, 0.0, 0.0, 0.0, 0.0, 0.0, 0.0, 0.0, 0.0, 0.0, 0.0, 0.0, 0.0, 0.0, 0.0, 0.0, 0.0, 0.0, 0.0, 0.0, 0.0, 0.0, 0.0, 0.0, 0.0, 0.0, 0.0, 0.0, 0.0, 0.0, 0.0, 0.0, 0.0, 0.0, 0.0, 0.0, 0.0, 0.0, 0.0, 0.0, 0.0, 0.0, 0.0, 0.0, 0.0, 0.0, 0.0, 0.0, 0.0, 0.0, 0.0, 0.0, 0.0, 0.0, 0.0, 0.0, 0.0, 0.0, 0.0, 0.0, 0.0, 0.0, 0.0, 0.0, 0.0, 0.0, 0.0, 0.0, 0.0, 0.0, 0.0, 0.0, 0.0, 0.0, 0.0, 0.0, 0.0, 0.0, 0.0, 0.0, 0.0, 0.0, 0.0, 0.0, 0.0, 0.0, 0.0, 0.0, 0.0, 0.0, 0.0, 0.0, 0.0, 0.0, 0.0, 0.0, 0.0, 0.0, 0.0, 0.0, 0.0, 0.0, 0.0, 0.0, 0.0, 0.0, 0.0, 0.0, 0.0, 0.0, 0.0, 0.0, 0.0, 0.0, 0.0, 0.0, 0.0, 0.0, 0.0, 0.0, 0.0, 0.0, 0.0, 0.0, 0.0, 0.0, 0.0, 0.0, 0.0, 0.0, 0.0, 0.0, 0.0, 0.0, 0.0, 0.0, 0.0, 0.0, 0.0, 0.0, 0.0, 0.0, 0.0, 0.0, 0.0, 0.0, 0.0, 0.0, 0.0, 0.0, 0.0, 0.0, 0.0, 0.0, 0.0, 0.0, 0.0, 0.0, 0.0, 0.0, 0.0, 0.0, 0.0, 0.0, 0.0, 0.0, 0.0, 0.0, 0.0, 0.0, 0.0, 0.0, 0.0, 0.0, 0.0, 0.0, 0.0, 0.0, 0.0, 0.0, 0.0, 0.0, 0.0, 0.0, 0.0, 0.0, 0.0, 0.0, 0.0, 0.0, 0.0, 0.0, 0.0, 0.0, 0.0, 0.0, 0.0, 0.0, 0.0, 0.0, 0.0, 0.0, 0.0, 0.0, 0.0, 0.0, 0.0, 0.0, 0.0, 0.0, 0.0, 0.0, 0.0, 0.0, 0.0, 0.0, 0.0, 0.0, 0.0, 0.0, 0.0, 0.0, 0.0, 0.0, 0.0, 0.0, 0.0, 0.0, 0.0, 0.0, 0.0, 0.0, 0.0, 0.0, 0.0, 0.0, 0.0, 0.0, 0.0, 0.0, 0.0, 0.0, 0.0, 0.0, 0.0, 0.0, 0.0, 0.0, 0.0, 0.0, 0.0, 0.0, 0.0, 0.0, 0.0, 0.0, 0.0, 0.0, 0.0, 0.0, 0.0, 0.0, 0.0, 0.0, 0.0, 0.0, 0.0, 0.0, 0.0, 0.0, 0.0, 0.0, 0.0, 0.0, 0.0, 0.0, 0.0, 0.0, 0.0, 0.0, 0.0, 0.0, 0.0, 0.0, 0.0, 0.0, 0.0, 0.0, 0.0, 0.0, 0.0, 0.0, 0.0, 0.0, 0.0, 0.0, 0.0, 0.0, 0.0, 0.0, 0.0, 0.0, 0.0, 0.0, 0.0, 0.0, 0.0, 0.0, 0.0, 0.0, 0.0, 0.0, 0.0, 0.0, 0.0, 0.0, 0.0, 0.0, 0.0, 0.0, 0.0, 0.0, 0.0, 0.0, 0.0, 0.0, 0.0, 0.0, 0.0, 0.0, 0.0, 0.0, 0.0, 0.0, 0.0, 0.0, 0.0, 0.0, 0.0, 0.0, 0.0, 0.0, 0.0, 0.0, 0.0, 0.0, 0.0, 0.0, 0.0, 0.0, 0.0, 0.0, 0.0, 0.0, 0.0, 0.0, 0.0, 0.0, 0.0, 0.0, 0.0, 0.0, 0.0, 0.0, 0.0, 0.0, 0.0, 0.0, 0.0, 0.0, 0.0, 0.0, 0.0, 0.0, 0.0, 0.0, 0.0, 0.0, 0.0, 0.0, 0.0, 0.0, 0.0, 0.0, 0.0, 0.0, 0.0, 0.0, 0.0, 0.0, 0.0, 0.0, 0.0, 0.0, 0.0, 0.0, 0.0, 0.0, 0.0, 0.0, 0.0, 0.0, 0.0, 0.0, 0.0, 0.0, 0.0, 0.0, 0.0, 0.0, 0.0, 0.0, 0.0, 0.0, 0.0, 0.0, 0.0, 0.0, 0.0, 0.0, 0.0, 0.0, 0.0, 0.0, 0.0, 0.0, 0.0, 0.0, 0.0, 0.0, 0.0, 0.0, 0.0, 0.0, 0.0, 0.0, 0.0, 0.0, 0.0, 0.0, 0.0, 0.0, 0.0, 0.0, 0.0, 0.0, 0.0, 0.0, 0.0, 0.0, 0.0, 0.0, 0.0, 0.0, 0.0, 0.0, 0.0, 0.0, 0.0, 0.0, 0.0, 0.0, 0.0, 0.0, 0.0, 0.0, 0.0, 0.0, 0.0, 0.0, 0.0, 0.0, 0.0, 0.0, 0.0, 0.0, 0.0, 0.0, 0.0, 0.0, 0.0, 0.0, 0.0, 0.0, 0.0, 0.0, 0.0, 0.0, 0.0, 0.0, 0.0, 0.0, 0.0, 0.0, 0.0, 0.0, 0.0, 0.0, 0.0, 0.0, 0.0, 0.0, 0.0, 0.0, 0.0, 0.0, 0.0, 0.0, 0.0, 0.0, 0.0, 0.0, 0.0, 0.0, 0.0, 0.0, 0.0, 0.0, 0.0, 0.0, 0.0, 0.0, 0.0, 0.0, 0.0, 0.0, 0.0, 0.0, 0.0, 0.0, 0.0, 0.0, 0.0, 0.0, 0.0, 0.0, 0.0, 0.0, 0.0, 0.0, 0.0, 0.0, 0.0, 0.0, 0.0, 0.0, 0.0, 0.0, 0.0, 0.0, 0.0, 0.0, 0.0, 0.0, 0.0, 0.0, 0.0, 0.0, 0.0, 0.0, 0.0, 0.0, 0.0, 0.0, 0.0, 0.0, 0.0, 0.0, 0.0, 0.0, 0.0, 0.0, 0.0, 0.0, 0.0, 0.0, 0.0, 0.0, 0.0, 0.0, 0.0, 0.0, 0.0, 0.0, 0.0, 0.0, 0.0, 0.0, 0.0, 0.0, 0.0, 0.0, 0.0, 0.0, 0.0, 0.0, 0.0, 0.0, 0.0, 0.0, 0.0, 0.0, 0.0, 0.0, 0.0, 0.0, 0.0, 0.0, 0.0, 0.0, 0.0, 0.0, 0.0, 0.0, 0.0, 0.0, 0.0, 0.0, 0.0, 0.0, 0.0, 0.0, 0.0, 0.0, 0.0, 0.0, 0.0, 0.0, 0.0, 0.0, 0.0, 0.0, 0.0, 0.0, 0.0, 0.0, 0.0, 0.0, 0.0, 0.0, 0.0, 0.0, 0.0, 0.0, 0.0, 0.0, 0.0, 0.0, 0.0, 0.0, 0.0, 0.0, 0.0, 0.0, 0.0, 0.0, 0.0, 0.0, 0.0, 0.0, 0.0, 0.0, 0.0, 0.0, 0.0, 0.0, 0.0, 0.0, 0.0, 0.0, 0.0, 0.0, 0.0, 0.0, 0.0, 0.0, 0.0, 0.0, 0.0, 0.0, 0.0, 0.0, 0.0, 0.0, 0.0, 0.0, 0.0, 0.0, 0.0, 0.0, 0.0, 0.0, 0.0, 0.0, 0.0, 0.0, 0.0, 0.0, 0.0, 0.0, 0.0, 0.0, 0.0, 0.0, 0.0, 0.0, 0.0, 0.0, 0.0, 0.0, 0.0, 0.0, 0.0, 0.0, 0.0, 0.0, 0.0, 0.0, 0.0, 0.0, 0.0, 0.0, 0.0, 0.0, 0.0, 0.0, 0.0, 0.0, 0.0, 0.0, 0.0, 0.0, 0.0, 0.0, 0.0, 0.0, 0.0, 0.0, 0.0, 0.0, 0.0, 0.0, 0.0, 0.0, 0.0, 0.0, 0.0, 0.0, 0.0, 0.0, 0.0, 0.0, 0.0, 0.0, 0.0, 0.0, 0.0, 0.0, 0.0, 0.0, 0.0, 0.0, 0.0, 0.0, 0.0, 0.0, 0.0, 0.0, 0.0, 0.0, 0.0, 0.0, 0.0, 0.0, 0.0, 0.0, 0.0, 0.0, 0.0, 0.0, 0.0, 0.0, 0.0, 0.0, 0.0, 0.0, 0.0, 0.0, 0.0, 0.0, 0.0, 0.0, 0.0, 0.0, 0.0, 0.0, 0.0, 0.0, 0.0, 0.0, 0.0, 0.0, 0.0, 0.0, 0.0, 0.0, 0.0, 0.0, 0.0] ("Data 2"), error in (no error)=errorcluster {"status"=FALSE, "code"=0, "source"=""} ("error constant")) -> (queue out=w17:refnum<queue>, error out=w16:errorcluster)  [unwired: 2 in, 1 out]
      n3 = xnode ("Open FPGA VI Reference")("error in"=w16, "resource name"=tag "rio://164.54.113.14/RIO0") -> ("FPGA VI Reference Out"=w24:refnum<k20>, "error out"=w25:errorcluster)
      n4 = shared-variable ".\\Interloop communication.lvlib\\Base Filename"(w22) -> ()  [unwired: 1 in, 1 out]
      n5 = shared-variable "RT CompactRIO Target\\RT_EPICS_Shared_Variables.lvlib\\2iddVELO:VP:Base_Filename"(w22) -> ()  [unwired: 1 in, 1 out]
      n6 = shared-variable "RT CompactRIO Target\\RT_EPICS_Shared_Variables.lvlib\\2iddVELO:VP:Remote_Scan"(TRUE ("Remote_Scan")) -> ()  [unwired: 1 in, 1 out]
      n7 = shared-variable "RT CompactRIO Target\\RT_EPICS_Shared_Variables.lvlib\\2iddVELO:VP:Fly_Scan"(FALSE ("Fly_Scan")) -> ()  [unwired: 1 in, 1 out]
      n8 = local write "Stop System (Careful!!)"(FALSE ("Stop")) -> ()
      n9 = shared-variable "RT CompactRIO Target\\RT_EPICS_Shared_Variables.lvlib\\2iddVELO:VP:Execute_Command"(w19) -> ()  [unwired: 1 in, 1 out]
      n10 = shared-variable "RT CompactRIO Target\\RT_EPICS_Shared_Variables.lvlib\\2iddVELO:VP:Scanning"(w19) -> ()  [unwired: 1 in, 1 out]
    }
  }
  n11 = node-c288() -> (w13:T12)  [unwired: 4 in]
  n12 = call <vilib>:"Clear Errors.vi"("error in (no error)"=w5) -> ("error out"=w2:errorcluster)  [unwired: 5 in, 1 out]
  n13 = while {
    tunnel: w6 -> [w32]
    tunnel: w5 -> [w31]
    i -> [w29]
    stop <- w30 stop-if-true
    # "Readback loop"
    n14 = local read "RT Main Loop State"() -> (w35:T10)
    n15 = Not Equal?(x=w35, y=State_Enum."Initialization") -> (x != y?=w33:bool)
    n16 = case shown="True" w33 {
      tunnel: w32 -> [_ w78]
      tunnel: w31 -> [_ w77]
      tunnel: [u32 100 ("milliseconds to wait") "Readback Loop time between iterations (ms)"] -> w28
      frame False {
      }
      frame True {
        w101 = 40000000.0  # FPGA Clock Rate (Hz)
        w48 = 40000000.0  # FPGA Clock Rate (Hz)
        w118 = 40000000.0  # FPGA Clock Rate (Hz)
        n17 = xnode "Read/Write Control"("FPGA VI Reference In"=w78, "error in"=w77) -> ("FPGA VI Reference Out"=w68:refnum<k20>, "error out"=w69:errorcluster, "FPGA state"=w74:T9, "Trajectory Complete"=→"Trajectory Completed":bool, "Run Loop error"=→"FPGA Run Loop error":errorcluster, "FPGA error monitor"=→"FPGA error monitor":errorcluster, "Stop Scan"=w44:bool)
        "FPGA state" <- w74
        n18 = local write "Stop Run"(w44) -> ()
        n19 = Format Into String(format string="%s", w74) -> (resulting string=w76:string)  [unwired: 2 in, 1 out]
        n20 = xnode ("Read/Write Control")("FPGA VI Reference In"=w68, "error in"=w69) -> ("error out"=w67:errorcluster, "Mod4/DIO0"=→"Mod4/DIO0":bool, "Mod4/DIO1"=→"Mod4/DIO1":bool, "Mod4/DIO2"=→"Mod4/DIO2":bool, "Mod4/DIO3"=→"Mod4/DIO3":bool, "Mod5/DIO0"=→"Mod5/DIO0":bool, "Mod5/DIO1"=→"Mod5/DIO1":bool, "Mod5/DIO2"=→"Mod5/DIO2":bool, "Mod5/DIO3"=→"Mod5/DIO3":bool, "Mod6/DIO0"=→"Mod6/DIO0":bool, "Mod6/DIO1"=→"Mod6/DIO1":bool, "Mod6/DIO2"=→"Mod6/DIO2":bool, "Mod6/DIO3"=→"Mod6/DIO3":bool, "Optics X Stage Displacement raw (nm)"=w53:fxp<+/-,32,16>, "Optics Y Stage Displacement raw (nm)"=w52:fxp<+/-,32,16>, "Optics Z Stage Displacement raw (nm)"=w51:fxp<+/-,32,16>, "Measured Datalog Period (Ticks)"=w57:u32, "Measured Counter Time Period (Ticks)"=w58:u32)  [unwired: 1 out]
        "Measured Datalog Time Period (Ticks)" <- w57
        "Measured Counter Time Period (Ticks)" <- w58
        "Optics X Stage Displacement (nm)" <- w53
        "Optics Y Stage Displacement (nm)" <- w52
        "Optics Z Stage Displacement (nm)" <- w51
        n21 = xnode ("Read/Write Control")("FPGA VI Reference In"=w68, "error in"=w69) -> ("error out"=w73:errorcluster, "Detector Trigger In Range?"=→"Detector Trigger In Range?":bool, "Number of Data Strings"=→"Number of Data Strings":i32, "Scan Type and Geometry"=→"Scan Type and Geometry":T11, "Position Number"=→"Position Number":u32, "Controller Output Lower Limit"=→"Controller Output Lower Limit Readback":fxp<+/-,20,5>, "Controller Output Upper Limit"=→"Controller Output Upper Limit Readback":fxp<+/-,20,5>, "Kxx Output, Kxx*ex (V)"=→"Kxx Output, Kxx*ex (V)":fxp<+/-,58,25>, "Kyy Output, Kyy*ey (V)"=→"Kyy Output, Kyy*ey (V)":fxp<+/-,58,25>, "Kzz Output, Kzz*ez (V)"=→"Kzz Output, Kzz*ez (V)":fxp<+/-,58,25>)  [unwired: 1 out]
        n22 = xnode "Read/Write Control"("FPGA VI Reference In"=w68, "error in"=w69) -> ("error out"=w66:errorcluster, "Controller loop iterations"=→"Controller loop iterations":i32, "Z Reference Loop iterations"=→"Z Reference Loop iterations":i32, "XY Reference Loop iterations"=→"XY Reference Loop iterations":i32, "FIFO loop iterations"=→"FIFO loop iterations":i32, "Trigger Generation Loop iterations"=→"Trigger Generation Loop iterations":i32, "Module output loop iterations"=→"Module output loop iterations":i32, "Plant output loop iterations"=→"Plant output loop iterations":i32, "Counter Loop iterations"=→"Counter Loop iterations":i32, "Outer Loop iterations"=→"Outer Loop iterations":i32)  [unwired: 1 out]
        n23 = xnode "Read/Write Control"("FPGA VI Reference In"=w68, "error in"=w69) -> ("error out"=w81:errorcluster, "X-Stage Input In Range?"=→"X-Stage Input In Range?":bool, "Y-Stage Input In Range?"=→"Y-Stage Input In Range?":bool, "Z-Stage Input In Range?"=→"Z-Stage Input In Range?":bool, "Measured Controller Loop Period (Ticks)"=w121:u32, "Measured Module Output Loop Period (Ticks)"=w120:u32, "Measured Plant Output Loop Period (Ticks)"=w119:u32)  [unwired: 1 out]
        "Measured Controller Time Period (Ticks)" <- w121
        "Measured Controller Output Time Period (Ticks)" <- w120
        "Measured Plant Output Time Period (Ticks)" <- w119
        n24 = xnode "Read/Write Control"("FPGA VI Reference In"=w68, "error in"=w69) -> ("error out"=w82:errorcluster, "Measured XY Reference Loop Period (ticks)"=w108:u32, "Measured Z Reference Loop Period (ticks)"=w105:u32, "Measured Trigger Generation Loop Period (Ticks)"=w47:u32)  [unwired: 1 out]
        "Measured XY Reference Time Period (Ticks)" <- w108
        "Measured Z Reference Time Period (Ticks)" <- w105
        "Measured Trigger Gen Time Period (Ticks)" <- w47
        n25 = shared-variable "RT CompactRIO Target\\RT_EPICS_Shared_Variables.lvlib\\2iddVELO:VP:FPGA_State"(w76) -> ()  [unwired: 1 in, 1 out]
        n26 = call "Convert Measured Rate.vi"("FPGA Clock Rate (Hz)"=w101, "Measured Reference Time Period (Ticks)"=w58) -> ("Measured Reference Loop Rate (kHz)"=w99:dbl, "Measured Reference Loop Period (us)"=→"Measured Counter Loop Rate (us)":dbl)
        n27 = call "Convert Measured Rate.vi"("FPGA Clock Rate (Hz)"=w101, "Measured Reference Time Period (Ticks)"=w57) -> ("Measured Reference Loop Rate (kHz)"=→"Measured Datalog Loop Rate (kHz)":dbl, "Measured Reference Loop Period (us)"=→"Measured Datalog Loop Rate (us)":dbl)
        n28 = call "Convert Measured Rate.vi"("FPGA Clock Rate (Hz)"=w118, "Measured Reference Time Period (Ticks)"=w121) -> ("Measured Reference Loop Rate (kHz)"=→"Measured Controller Loop Rate (kHz)":dbl, "Measured Reference Loop Period (us)"=→"Measured Controller Loop Rate (us)":dbl)
        n29 = call "Convert Measured Rate.vi"("FPGA Clock Rate (Hz)"=w118, "Measured Reference Time Period (Ticks)"=w120) -> ("Measured Reference Loop Rate (kHz)"=→"Measured Controller Output Loop Rate (kHz)":dbl, "Measured Reference Loop Period (us)"=→"Measured Controller Output Loop Rate (us)":dbl)
        n30 = call "Convert Measured Rate.vi"("FPGA Clock Rate (Hz)"=w118, "Measured Reference Time Period (Ticks)"=w119) -> ("Measured Reference Loop Rate (kHz)"=→"Measured Plant Output Loop Rate (kHz)":dbl, "Measured Reference Loop Period (us)"=→"Measured Plant Output Loop Rate (us)":dbl)
        n31 = call "Convert Measured Rate.vi"("FPGA Clock Rate (Hz)"=w48, "Measured Reference Time Period (Ticks)"=w47) -> ("Measured Reference Loop Rate (kHz)"=→"Measured Trigger Gen Loop Rate (kHz)":dbl, "Measured Reference Loop Period (us)"=→"Measured Trigger Gen Loop Rate (us)":dbl)
        n32 = call "Convert Measured Rate.vi"("FPGA Clock Rate (Hz)"=w48, "Measured Reference Time Period (Ticks)"=w105) -> ("Measured Reference Loop Rate (kHz)"=→"Measured Z Reference Loop Rate (kHz)":dbl, "Measured Reference Loop Period (us)"=→"Measured Z Reference Loop Rate (us)":dbl)
        n33 = call "Convert Measured Rate.vi"("FPGA Clock Rate (Hz)"=w48, "Measured Reference Time Period (Ticks)"=w108) -> ("Measured Reference Loop Rate (kHz)"=→"Measured XY Reference Loop Rate (kHz)":dbl, "Measured Reference Loop Period (us)"=→"Measured XY Reference Loop Rate (us)":dbl)
        n34 = Divide(x=w99, y=1000.0) -> (x/y=→"Measured Counter Loop Rate (MHz)":dbl)
        n35 = To Double Precision Float(number=w51) -> (double precision float=w54:dbl)
        n36 = To Double Precision Float(number=w53) -> (double precision float=w56:dbl)
        n37 = To Double Precision Float(number=w52) -> (double precision float=w55:dbl)
        n38 = shared-variable "RT CompactRIO Target\\RT_EPICS_Shared_Variables.lvlib\\2iddVELO:LabView:ZPY_Readback"(w55) -> ()  [unwired: 1 in, 1 out]
        n39 = shared-variable "RT CompactRIO Target\\RT_EPICS_Shared_Variables.lvlib\\2iddVELO:LabView:ZPX_Readback"(w56) -> ()  [unwired: 1 in, 1 out]
        n40 = shared-variable "RT CompactRIO Target\\RT_EPICS_Shared_Variables.lvlib\\2iddVELO:LabView:ZPZ_Readback"(w54) -> ()  [unwired: 1 in, 1 out]
        n41 = Merge Errors(w81, w82, w73, w66, w67) -> (w80:errorcluster)
        "Readback error" <- w80
        n42 = shared-variable ".\\Interloop communication.lvlib\\Readback Loop Error"(w80) -> ()  [unwired: 1 in, 1 out]
      }
    }
    n43 = local read "Stop System (Careful!!)"() -> (w30:bool)
    n44 = Wait (ms)(milliseconds to wait=w28) -> ()  [unwired: 1 out]
    "Readback loop Iterations" <- w29
  }
  n45 = while {
    i -> [w123]
    stop <- w124 stop-if-true
    # "Command  Loop"
    n46 = Wait Until Next ms Multiple(millisecond multiple=u32 50) -> ()  [unwired: 1 out]
    n47 = case shown="False" "Stop System (Careful!!)" {
      tunnel: [FALSE TRUE] -> w124
      frame False {
        n48 = shared-variable "RT CompactRIO Target\\RT_EPICS_Shared_Variables.lvlib\\2iddVELO:VP:Remote_Scan"() -> (w135:bool, error out=w133:errorcluster)  [unwired: 1 in]
        n49 = shared-variable "RT CompactRIO Target\\RT_EPICS_Shared_Variables.lvlib\\2iddVELO:VP:Local_Lock"("Local_Lock", error in=w133) -> (error out=w128:errorcluster)
        n50 = shared-variable ".\\Interloop communication.lvlib\\New Command"() -> (w138:bool)  [unwired: 1 in, 1 out]
        n51 = Not(x="Local_Lock") -> (.not. x?=w130:bool)
        n52 = And(x=w135, y=w130) -> (x .and. y?=w136:bool)
        "Remote Mode" <- w136
        n53 = Not(x=w138) -> (.not. x?=w137:bool)
        n54 = case shown="False" w136 {
          tunnel: w137 -> [w148 w160]
          tunnel: [Local_or_Remote."Local Control" ("Local or EPICS") Local_or_Remote."EPICS Control" ("Local or EPICS")] -> w127
          tunnel: w128 -> [w142 w155]
          tunnel: [w144 w158] -> w132
          tunnel: ["Base name" w157] -> w129
          frame False {
            # "Running  in local mode"
            n55 = And(x="Execute", y=w148) -> (x .and. y?=w146:bool)
            n56 = case shown="True" w146 {
              frame False {
              }
              frame True {
                n57 = shared-variable ".\\Interloop communication.lvlib\\New Command"(TRUE ("New Command")) -> ()  [unwired: 1 in, 1 out]
                n58 = shared-variable ".\\Interloop communication.lvlib\\System command"("System command") -> ()  [unwired: 1 in, 1 out]
                n59 = local write "Execute"(FALSE ("Execute")) -> ()
              }
            }
            n60 = Format Into String(error in=w142, "Scan type") -> (resulting string=w143:string, error out=w141:errorcluster)  [unwired: 2 in]
            n61 = shared-variable "RT CompactRIO Target\\RT_EPICS_Shared_Variables.lvlib\\2iddVELO:VP:Scan_Type"(w143, error in=w141) -> (error out=w144:errorcluster)
          }
          frame True {
            # "Running in remote mode via EPICS PVs"
            n62 = shared-variable "RT CompactRIO Target\\RT_EPICS_Shared_Variables.lvlib\\2iddVELO:VP:Execute_Command"(error in=w155) -> (w156:bool, error out=w154:errorcluster)
            "EPICS Execute Command" <- w156
            n63 = shared-variable "RT CompactRIO Target\\RT_EPICS_Shared_Variables.lvlib\\2iddVELO:VP:Base_Filename"() -> (w157:string)  [unwired: 1 in, 1 out]
            n64 = And(x=w160, y=w156) -> (x .and. y?=w159:bool)
            n65 = case shown="True" w159 {
              tunnel: [w161 w169] -> w158
              tunnel: w154 -> [w161 w166]
              frame False {
              }
              frame True {
                n66 = local read "EPICS cRIO Command"() -> (w167:T5)
                n67 = local read "EPICS Scan Trajectory"() -> (w162:T3)
                n68 = local read "EPICS Scan Type"() -> (w163:enum16{"Fly", "Step"})
                n69 = shared-variable "RT CompactRIO Target\\RT_EPICS_Shared_Variables.lvlib\\2iddVELO:VP:Execute_Command"(FALSE ("2iddVELO:VP:Flyscan_Start"), error in=w166) -> (error out=w169:errorcluster)
                n70 = shared-variable ".\\Interloop communication.lvlib\\New Command"(TRUE ("New Command")) -> ()  [unwired: 1 in, 1 out]
                n71 = case shown="\"Stop Scan\"" w167 {
                  tunnel: [Command_Enum."Scan" ("System command") Command_Enum."Stop Scan" ("System command") Command_Enum."Re-Initialize " ("System command")] -> w164
                  frame "Start Scan", Default {
                  }
                  frame "Stop Scan" {
                  }
                  frame "Reload Controller" {
                  }
                }
                n72 = local write "Scan type"(w163) -> ()
                n73 = local write "Scan Geometry"(w162) -> ()
                n74 = shared-variable ".\\Interloop communication.lvlib\\System command"(w164) -> ()  [unwired: 1 in, 1 out]
                n75 = local write "System Loop Type"(enum16{"Open Loop", "Closed Loop"}."Closed Loop" ("System Loop Type")) -> ()
              }
            }
            n76 = local write "Base name"(w157) -> ()
            n77 = local read "EPICS Controller Type"() -> (w153:T2)
            n78 = local write "Controller Type"(w153) -> ()
          }
        }
        "Local or EPICS" <- w127
        "Command Loop Error" <- w132
        n79 = shared-variable ".\\Interloop communication.lvlib\\Base Filename"(w129) -> ()  [unwired: 1 in, 1 out]
        n80 = shared-variable ".\\Interloop communication.lvlib\\Command Loop Error"(w132) -> ()  [unwired: 1 in, 1 out]
      }
      frame True {
        n81 = shared-variable ".\\Interloop communication.lvlib\\System command"(Command_Enum."Stop System" ("System command")) -> (error out=w174:errorcluster)  [unwired: 1 in]
        n82 = shared-variable ".\\Interloop communication.lvlib\\New Command"(TRUE ("New Command"), error in=w174) -> ()  [unwired: 1 out]
      }
    }
    "Command Loop Iterations" <- w123
  }
  n83 = timed-loop {
    timing: w13 -> [_]
    timing-out: [_] -> w12
    shift-right: [w190] -> _
    shift-left: w8 -> [w184]
    shift-right: [w197] -> _
    shift-left: w6 -> [w191]
    shift-right: [w188] -> w4
    shift-left: w5 -> [w192]
    shift-right: [w194] -> _
    shift-left: w7 -> [w195]
    tunnel: w3 -> [w182]
    shift-right: [w179] -> _
    shift-left: FALSE -> [w180]
    i -> [w196]
    stop <- w199 stop-if-true
    # "Main Loop"
    n84 = node-c288() -> (→"Iteration Duration":i64)  [unwired: 1 in, 1 out]
    n85 = Format Into String(format string="%s", w184) -> (resulting string=w185:string)  [unwired: 2 in, 1 out]
    n86 = shared-variable "RT CompactRIO Target\\RT_EPICS_Shared_Variables.lvlib\\2iddVELO:VP:RT_State"(w185) -> ()  [unwired: 1 in, 1 out]
    n87 = local read "Local or EPICS"() -> (w189:T8)
    n88 = local read "Scan Geometry"() -> (w178:T3)
    n89 = local read "Scan type"() -> (w183:enum16{"Fly", "Step"})
    n90 = case shown="\"Restart FPGA\"" w184 {
      tunnel: [w207 w220 w261 w317 w377 w453 w480 w492 w519 w576 w600 w623 w649 w673 w700 w713] -> w198
      tunnel: [FALSE ("Stop") FALSE ("Stop") FALSE ("Stop") FALSE ("Stop") FALSE ("Stop") FALSE ("Stop") FALSE ("Stop") FALSE ("Stop") _ FALSE ("Stop") FALSE ("Stop") FALSE ("Stop") FALSE ("Stop") FALSE ("Stop") FALSE ("Stop") TRUE ("Stop")] -> w199
      tunnel: [w208 w225 w260 w319 w376 w452 w479 w494 w510 w567 w593 w617 w650 w669 w695 w710] -> w197
      tunnel: [w204 w222 w259 w313 w375 w451 w478 w485 w509 w566 w592 w637 w647 w674 w694 w715] -> w188
      tunnel: w192 -> [w201 w217 w263 w314 w366 w446 w481 w495 w517 w571 w594 w620 w654 w670 w698 w719]
      tunnel: w191 -> [w202 w225 w262 w319 w378 w454 w482 w496 w518 w572 w595 w639 w656 w669 w704 w720]
      tunnel: w195 -> [w207 w220 w261 _ w377 w453 w480 w492 w519 w576 w601 w624 w649 w672 w700 _]
      tunnel: [i64 0 i64 0 i64 0 i64 50 i64 0 i64 0 i64 0 i64 0 i64 0 "Start Scan Loop dt" i64 50 "Fly scan loop dt" i64 0 i64 0 i64 0 i64 0] -> w193
      tunnel: w189 -> [_ _ _ _ w372 w448 _ _ _ _ w588 _ _ _ _ _]
      tunnel: w183 -> [_ _ _ w311 w353 _ _ _ w504 w569 _ _ w651 _ _ _]
      tunnel: w182 -> [_ _ _ _ _ _ _ _ _ _ _ w618 _ _ _ _]
      tunnel: w180 -> [_ _ _ _ _ _ _ _ _ _ _ w613 _ _ _ _]
      tunnel: [FALSE FALSE FALSE FALSE FALSE FALSE FALSE FALSE FALSE FALSE FALSE TRUE FALSE FALSE FALSE FALSE] -> w179
      tunnel: w178 -> [_ _ _ _ w354 _ _ _ _ _ _ _ _ _ _ _]
      frame "Initialization", Default {
        n91 = xnode "Read/Write Control"("FPGA VI Reference In"=w202, "error in"=w201) -> ("FPGA VI Reference Out"=w208:refnum<k20>, "error out"=w204:errorcluster, "Wait error"=w203:errorcluster)
        "FPGA wait error" <- w203
        n92 = shared-variable ".\\Interloop communication.lvlib\\FPGA startup error"(w203) -> ()  [unwired: 1 in, 1 out]
      }
      frame "Import Controller coeffs" {
        n93 = case shown="\"PID\"" "Controller Type" {
          tunnel: ["file path soscoeff_xx1 Hinf" "file path soscoeff_xx1 PID"] -> w216
          tunnel: ["file path sos gain SF Controller_xx1 Hinf" "file path sos gain SF Controller_xx1 PID"] -> w215
          tunnel: ["file path soscoeff_yy1 Hinf" "file path soscoeff_yy1 PID"] -> w214
          tunnel: ["file path sos gain SF Controller_yy1 Hinf" "file path sos gain SF Controller_yy1 PID"] -> w213
          tunnel: ["file path sos gain SF Controller_zz1 Hinf" "file path sos gain SF Controller_zz1 PID"] -> w212
          tunnel: ["file path soscoeff_zz1 Hinf" "file path soscoeff_zz1 PID"] -> w211
          frame "H-infinity", Default {
          }
          frame "PID" {
          }
        }
        n94 = call "Read_coeff.vi"("error in (no error)"=w217, "sos gain SF controller file path"=w215, "sos coeff file path"=w216) -> ("b02(2)"=→"b02(2) xx1c":fxp<+/-,64,9>[], "b01(2)"=→"b01(2) xx1c":fxp<+/-,64,9>[], "-a02(2)"=→"-a02(2) xx1c":fxp<+/-,64,9>[], "-a01(2)"=→"-a01(2) xx1c":fxp<+/-,64,9>[], "error out"=w218:errorcluster, "sos gain SF Controller"=→"sos gain SF Controller xx1c":fxp<+/-,42,9>)  [unwired: 3 in]
        n95 = call "Read_coeff.vi"("error in (no error)"=w217, "sos gain SF controller file path"=w213, "sos coeff file path"=w214) -> ("b02(2)"=→"b02(2) yy1c":fxp<+/-,64,9>[], "b01(2)"=→"b01(2) yy1c":fxp<+/-,64,9>[], "-a02(2)"=→"-a02(2) yy1c":fxp<+/-,64,9>[], "-a01(2)"=→"-a01(2) yy1c":fxp<+/-,64,9>[], "error out"=w219:errorcluster, "sos gain SF Controller"=→"sos gain SF Controller yy1c":fxp<+/-,42,9>)  [unwired: 3 in]
        n96 = call "Read_coeff.vi"("error in (no error)"=w217, "sos gain SF controller file path"=w212, "sos coeff file path"=w211) -> ("b02(2)"=→"b02(2) zz1c":fxp<+/-,64,9>[], "b01(2)"=→"b01(2) zz1c":fxp<+/-,64,9>[], "-a02(2)"=→"-a02(2) zz1c":fxp<+/-,64,9>[], "-a01(2)"=→"-a01(2) zz1c":fxp<+/-,64,9>[], "error out"=w221:errorcluster, "sos gain SF Controller"=→"sos gain SF Controller zz1c":fxp<+/-,42,9>)  [unwired: 3 in]
        n97 = Merge Errors(w218, w219, w221) -> (w222:errorcluster)
        "Coeff file import error" <- w222
      }
      frame "Update Controller Info" {
        n98 = local read "sos gain SF Controller yy1c"() -> (w291:fxp<+/-,42,9>)
        n99 = local read "sos gain SF Controller xx1c"() -> (w296:fxp<+/-,42,9>)
        n100 = local read "sos gain SF Controller zz1c"() -> (w289:fxp<+/-,42,9>)
        n101 = local read "-a01(2) yy1c"() -> (w295:fxp<+/-,64,9>[])
        n102 = local read "-a02(2) yy1c"() -> (w294:fxp<+/-,64,9>[])
        n103 = local read "-a01(2) xx1c"() -> (w300:fxp<+/-,64,9>[])
        n104 = local read "-a02(2) xx1c"() -> (w299:fxp<+/-,64,9>[])
        n105 = local read "-a01(2) zz1c"() -> (w290:fxp<+/-,64,9>[])
        n106 = local read "-a02(2) zz1c"() -> (w286:fxp<+/-,64,9>[])
        n107 = local read "b01(2) yy1c"() -> (w293:fxp<+/-,64,9>[])
        n108 = local read "b02(2) yy1c"() -> (w292:fxp<+/-,64,9>[])
        n109 = local read "b01(2) xx1c"() -> (w298:fxp<+/-,64,9>[])
        n110 = local read "b02(2) xx1c"() -> (w297:fxp<+/-,64,9>[])
        n111 = local read "b01(2) zz1c"() -> (w287:fxp<+/-,64,9>[])
        n112 = local read "b02(2) zz1c"() -> (w288:fxp<+/-,64,9>[])
        n113 = Or(x="Optics Z Reset", y="Reset All") -> (x .or. y?=w280:bool)
        n114 = Or(x="Sample Z Reset", y="Reset All") -> (x .or. y?=w277:bool)
        n115 = Or(x="Optics X Reset", y="Reset All") -> (x .or. y?=w284:bool)
        n116 = Or(x="Optics Y Reset", y="Reset All") -> (x .or. y?=w282:bool)
        n117 = Or(x="Sample X Reset", y="Reset All") -> (x .or. y?=w279:bool)
        n118 = Or(x="Sample Y Reset", y="Reset All") -> (x .or. y?=w278:bool)
        n119 = xnode "Read/Write Control"("FPGA VI Reference In"=w262, "error in"=w263, "Wait timer (ms)"="FPGA Wait Timer (ms)", "Controller Loop Period (uSec)"="Controller Time Period (uSec)", "Module Output Loop Period (uSec)"="Controller Output Time Period (uSec)", "System Loop Type"="System Loop Type", "Controller Output Upper Limit"="Controller Output Upper Limit", "Controller Output Lower Limit"="Controller Output Lower Limit", "X-Stage nm to V Scaling"="X-Stage nm to V Scaling", "X-Stage Scaling Direction"="X-Stage Scaling Direction", "Y-Stage nm to V Scaling"="Y-Stage nm to V Scaling", "Z-Stage nm to V Scaling"="Z-Stage nm to V Scaling", "Plant Output Loop Period (uSec)"="Plant Output Time Period (uSec)", "Reset Optics X"=w284, "Reset Optics Y"=w282, "Reset Optics Z"=w280, "Reset Sample X"=w279, "Reset Sample Y"=w278, "Reset Sample Z"=w277, "Optics X Stage Resolution (nm)"="Optics X Stage Resolution (nm)", "Optics Y Stage Resolution (nm)"="Optics Y Stage Resolution (nm)", "Optics Z Stage Resolution (nm)"="Optics Z Stage Resolution (nm)", "Sample X Stage Resolution (nm)"="Sample X Stage Resolution (nm)", "Sample Y Stage Resolution (nm)"="Sample Y Stage Resolution (nm)", "Sample Z Stage Resolution (nm)"="Sample Z Stage Resolution (nm)", "Scaling mV to V"="Scaling mV to V", "-a01(2) xx1"=w300, "-a02(2) xx1"=w299, "b01(2) xx1"=w298, "b02(2) xx1"=w297, "sos gain SF Controller xx1"=w296, "-a01(2) yy1"=w295, "-a02(2) yy1"=w294, "b01(2) yy1"=w293, "b02(2) yy1"=w292, "sos gain SF Controller yy1"=w291, "-a01(2) zz1"=w290, "-a02(2) zz1"=w286, "b01(2) zz1"=w287, "b02(2) zz1"=w288, "sos gain SF Controller zz1"=w289, "Optics and or Sample Stage"="Optics and or Sample Stage", "Y-Stage Scaling Direction"="Y-Stage Scaling Direction", "Z-Stage Scaling Direction"="Z-Stage Scaling Direction") -> ("FPGA VI Reference Out"=w260:refnum<k20>, "error out"=w259:errorcluster)
      }
      frame "Wait" {
        n120 = shared-variable ".\\Interloop communication.lvlib\\New Command"() -> (w318:bool, error out=w316:errorcluster)  [unwired: 1 in]
        n121 = case shown="True" w318 {
          tunnel: [w321 w323] -> w317
          tunnel: w316 -> [_ w327]
          tunnel: w314 -> [w320 w325]
          tunnel: [w320 w324] -> w313
          tunnel: w311 -> [_ w322]
          frame False {
            w321 = T10[] [enum."Wait"] items=["Initialization", "Import Controller coeffs", "Update Controller Info", "Wait", "Update Reference Info", "Update Detector Trigger Info", "Update Datalog Info", "Check FPGA Status", "Initialize FIFO", "Pre-Scan", "Start Scan", "Step Scanning", "Fly Scanning", "End Scan", "Close File", "Restart FPGA", "Stop FPGA"]
          }
          frame True {
            n122 = shared-variable ".\\Interloop communication.lvlib\\System command"() -> (w326:T6)  [unwired: 1 in, 1 out]
            "Last Command Executed" <- w326
            n123 = case shown="\"Scan\"" w326 {
              tunnel: [w331 w334 w338 w343 w346 w350] -> w323
              tunnel: w325 -> [w330 w333 w337 w342 w345 w349]
              tunnel: [w329 w332 w336 w341 w344 w348] -> w324
              tunnel: w322 -> [_ _ w335 _ _ _]
              frame "Re-Initialize ", Default {
                w331 = T10[] [enum."Initialization", enum."Import Controller coeffs", enum."Update Controller Info", enum."Wait"] items=["Initialization", "Import Controller coeffs", "Update Controller Info", "Wait", "Update Reference Info", "Update Detector Trigger Info", "Update Datalog Info", "Check FPGA Status", "Initialize FIFO", "Pre-Scan", "Start Scan", "Step Scanning", "Fly Scanning", "End Scan", "Close File", "Restart FPGA", "Stop FPGA"]
                n124 = call <vilib>:"Clear Errors.vi"("error in (no error)"=w330) -> ("error out"=w329:errorcluster)  [unwired: 5 in, 1 out]
              }
              frame "Update Scan Settings" {
                w334 = T10[] [enum."Update Reference Info", enum."Update Detector Trigger Info", enum."Update Datalog Info", enum."Wait"] items=["Initialization", "Import Controller coeffs", "Update Controller Info", "Wait", "Update Reference Info", "Update Detector Trigger Info", "Update Datalog Info", "Check FPGA Status", "Initialize FIFO", "Pre-Scan", "Start Scan", "Step Scanning", "Fly Scanning", "End Scan", "Close File", "Restart FPGA", "Stop FPGA"]
                n125 = call <vilib>:"Clear Errors.vi"("error in (no error)"=w333) -> ("error out"=w332:errorcluster)  [unwired: 5 in, 1 out]
              }
              frame "Scan" {
                n126 = case shown="\"Step\"" w335 {
                  tunnel: [w339 w340] -> w338
                  frame "Fly", Default {
                    w339 = T10[] [enum."Update Reference Info", enum."Update Detector Trigger Info", enum."Update Datalog Info", enum."Pre-Scan", enum."Start Scan", enum."Fly Scanning", enum."End Scan", enum."Close File", enum."Wait"] items=["Initialization", "Import Controller coeffs", "Update Controller Info", "Wait", "Update Reference Info", "Update Detector Trigger Info", "Update Datalog Info", "Check FPGA Status", "Initialize FIFO", "Pre-Scan", "Start Scan", "Step Scanning", "Fly Scanning", "End Scan", "Close File", "Restart FPGA", "Stop FPGA"]
                  }
                  frame "Step" {
                    w340 = T10[] [enum."Update Reference Info", enum."Update Detector Trigger Info", enum."Update Datalog Info", enum."Pre-Scan", enum."Start Scan", enum."Step Scanning", enum."End Scan", enum."Wait"] items=["Initialization", "Import Controller coeffs", "Update Controller Info", "Wait", "Update Reference Info", "Update Detector Trigger Info", "Update Datalog Info", "Check FPGA Status", "Initialize FIFO", "Pre-Scan", "Start Scan", "Step Scanning", "Fly Scanning", "End Scan", "Close File", "Restart FPGA", "Stop FPGA"]
                  }
                }
                n127 = call <vilib>:"Clear Errors.vi"("error in (no error)"=w337) -> ("error out"=w336:errorcluster)  [unwired: 5 in, 1 out]
              }
              frame "Stop Scan" {
                w343 = T10[] [enum."End Scan", enum."Wait"] items=["Initialization", "Import Controller coeffs", "Update Controller Info", "Wait", "Update Reference Info", "Update Detector Trigger Info", "Update Datalog Info", "Check FPGA Status", "Initialize FIFO", "Pre-Scan", "Start Scan", "Step Scanning", "Fly Scanning", "End Scan", "Close File", "Restart FPGA", "Stop FPGA"]
                n128 = call <vilib>:"Clear Errors.vi"("error in (no error)"=w342) -> ("error out"=w341:errorcluster)  [unwired: 5 in, 1 out]
              }
              frame "Restart FPGA" {
                w346 = T10[] [enum."Restart FPGA", enum."Initialization", enum."Import Controller coeffs", enum."Update Controller Info", enum."Wait"] items=["Initialization", "Import Controller coeffs", "Update Controller Info", "Wait", "Update Reference Info", "Update Detector Trigger Info", "Update Datalog Info", "Check FPGA Status", "Initialize FIFO", "Pre-Scan", "Start Scan", "Step Scanning", "Fly Scanning", "End Scan", "Close File", "Restart FPGA", "Stop FPGA"]
                n129 = call <vilib>:"Clear Errors.vi"("error in (no error)"=w345) -> ("error out"=w344:errorcluster)  [unwired: 5 in, 1 out]
              }
              frame "Stop System" {
                w350 = T10[] [enum."Stop FPGA"] items=["Initialization", "Import Controller coeffs", "Update Controller Info", "Wait", "Update Reference Info", "Update Detector Trigger Info", "Update Datalog Info", "Check FPGA Status", "Initialize FIFO", "Pre-Scan", "Start Scan", "Step Scanning", "Fly Scanning", "End Scan", "Close File", "Restart FPGA", "Stop FPGA"]
                n130 = call <vilib>:"Clear Errors.vi"("error in (no error)"=w349) -> ("error out"=w348:errorcluster)  [unwired: 5 in, 1 out]
                n131 = local write "Stop System (Careful!!)"(TRUE ("Stop")) -> ()
              }
            }
            n132 = shared-variable ".\\Interloop communication.lvlib\\New Command"(FALSE ("New Command"), error in=w327) -> ()  [unwired: 1 out]
          }
        }
      }
      frame "Update Reference Info" {
        w392 = 40000000.0  # FPGA clock rate (Hz)
        n133 = case shown="\"EPICS Control\"" w372 {
          tunnel: ["X Step Size (nm)" w427] -> w363
          tunnel: [w409 w426] -> w379
          tunnel: ["Y Step Size (nm)" w425] -> w368
          tunnel: ["X Ramp Start (nm)" w424] -> w370
          tunnel: ["X Ramp End (nm)" w423] -> w364
          tunnel: ["Y Ramp Start (nm)" w422] -> w362
          tunnel: ["Y Ramp End (nm)" w421] -> w369
          tunnel: ["Spiral Step Size" w418] -> w361
          tunnel: ["Max radius" w417] -> w360
          tunnel: ["Radial direction" w414] -> w357
          tunnel: ["Rotation Direction" w413] -> w356
          tunnel: ["Inner Scan axis" w412] -> w355
          tunnel: w354 -> [_ w411]
          frame "Local Control", Default {
            n134 = local read "DT Frequency (Hz)"() -> (w409:dbl)
          }
          frame "EPICS Control" {
            n135 = shared-variable "RT CompactRIO Target\\RT_EPICS_Shared_Variables.lvlib\\2iddVELO:VP:Trigger_Freq_Hz"() -> (w426:dbl)  [unwired: 1 in, 1 out]
            "2iddVELO:VP:Trigger_Freq_Hz" <- w426
            n136 = shared-variable "RT CompactRIO Target\\RT_EPICS_Shared_Variables.lvlib\\2iddVELO:VP:Y_Step_Size_nm"() -> (w429:dbl)  [unwired: 1 in, 1 out]
            "2iddVELO:VP:Y_Step_Size_nm" <- w429
            n137 = shared-variable "RT CompactRIO Target\\RT_EPICS_Shared_Variables.lvlib\\2iddVELO:VP:X_Step_Size_nm"() -> (w428:dbl)  [unwired: 1 in, 1 out]
            "2iddVELO:VP:X_Step_Size_nm" <- w428
            n138 = case shown="\"Archimedes Spiral\", Default" w411 {
              tunnel: [w439 w442] -> w424
              tunnel: [w438 w441] -> w422
              frame "Archimedes Spiral", Default {
                n139 = shared-variable "RT CompactRIO Target\\RT_EPICS_Shared_Variables.lvlib\\2iddVELO:VP:Y_Center"() -> (w434:dbl)  [unwired: 1 in, 1 out]
                n140 = shared-variable "RT CompactRIO Target\\RT_EPICS_Shared_Variables.lvlib\\2iddVELO:VP:X_Center"() -> (w437:dbl)  [unwired: 1 in, 1 out]
                "2iddVELO:VP:X_Center" <- w437
                n141 = Negate(x=w434) -> (-x=w433:dbl)
                "2iddVELO:VP:Y_Center" <- w433
                n142 = Multiply(x=w437, y=1000.0) -> (x*y=w436:dbl)
                n143 = Multiply(x=w433, y=1000.0) -> (x*y=w431:dbl)
                n144 = To Fixed-Point(number=w431) -> (fixed-point=w438:fxp<+/-,32,16>)  [unwired: 1 in]
                n145 = To Fixed-Point(number=w436) -> (fixed-point=w439:fxp<+/-,32,16>)  [unwired: 1 in]
              }
              frame "Grid Spiral", "Snake" {
                n146 = shared-variable "RT CompactRIO Target\\RT_EPICS_Shared_Variables.lvlib\\2iddVELO:VP:Y_Start_nm"() -> (w443:dbl)  [unwired: 1 in, 1 out]
                n147 = shared-variable "RT CompactRIO Target\\RT_EPICS_Shared_Variables.lvlib\\2iddVELO:VP:X_Start_nm"() -> (w444:dbl)  [unwired: 1 in, 1 out]
                "2iddVELO:VP:X_Start_nm" <- w444
                n148 = Negate(x=w443) -> (-x=w440:dbl)
                "2iddVELO:VP:Y_Start_nm" <- w440
                n149 = To Fixed-Point(number=w440) -> (fixed-point=w441:fxp<+/-,32,16>)  [unwired: 1 in]
                n150 = To Fixed-Point(number=w444) -> (fixed-point=w442:fxp<+/-,32,16>)  [unwired: 1 in]
              }
            }
            n151 = shared-variable "RT CompactRIO Target\\RT_EPICS_Shared_Variables.lvlib\\2iddVELO:VP:Max_Radius"() -> (w415:dbl)  [unwired: 1 in, 1 out]
            "2iddVELO:VP:Max_Radius" <- w415
            n152 = shared-variable "RT CompactRIO Target\\RT_EPICS_Shared_Variables.lvlib\\2iddVELO:VP:Spiral_Step"() -> (w416:dbl)  [unwired: 1 in, 1 out]
            "2iddVELO:VP:Spiral_Step" <- w416
            n153 = shared-variable "RT CompactRIO Target\\RT_EPICS_Shared_Variables.lvlib\\2iddVELO:VP:X_End_nm"() -> (w430:dbl)  [unwired: 1 in, 1 out]
            "2iddVELO:VP:X_End_nm" <- w430
            n154 = shared-variable "RT CompactRIO Target\\RT_EPICS_Shared_Variables.lvlib\\2iddVELO:VP:Y_End_nm"() -> (w420:dbl)  [unwired: 1 in, 1 out]
            n155 = Negate(x=w420) -> (-x=w419:dbl)
            "2iddVELO:VP:Y_End_nm" <- w419
            n156 = local read "EPICS rotation direction"() -> (w413:enum16{"Clockwise", "Anti-clockwise"})
            n157 = local read "EPICS radial direction"() -> (w414:enum16{"Outward", "Inward"})
            n158 = To Fixed-Point(number=w430) -> (fixed-point=w423:fxp<+/-,32,16>)  [unwired: 1 in]
            n159 = To Fixed-Point(number=w419) -> (fixed-point=w421:fxp<+/-,32,16>)  [unwired: 1 in]
            n160 = To Fixed-Point(number=w429) -> (fixed-point=w425:fxp<+/-,32,16>)  [unwired: 1 in]
            n161 = To Fixed-Point(number=w428) -> (fixed-point=w427:fxp<+/-,32,16>)  [unwired: 1 in]
            n162 = local read "EPICS Inner axis"() -> (w412:enum16{"X", "Y"})
            n163 = To Fixed-Point(number=w416) -> (fixed-point=w418:fxp<+/-,32,16>)  [unwired: 1 in]
            n164 = To Fixed-Point(number=w415) -> (fixed-point=w417:fxp<+/-,32,16>)  [unwired: 1 in]
          }
        }
        n165 = call <vilib>:"Normalize Signal Generation Parameters.vi"("frequency (Hz)"="Trajectory frequency (Hz)", "FPGA clock rate (Hz)"=w392, "error in (no error)"=w366) -> ("frequency (periods/tick)"=w371:fxp<+,32,0>, "actual frequency (Hz)"=→"actual Traj frequency (Hz)":dbl, "error out"=w365:errorcluster)  [unwired: 7 in, 3 out]
        "Trajectory frequency (periods/tick)" <- w371
        n166 = Subtract(x=w362, y=w369) -> (x-y=w389:fxp<+/-,33,17>)
        n167 = Subtract(x=w370, y=w364) -> (x-y=w387:fxp<+/-,33,17>)
        n168 = Absolute Value(x=w389) -> (abs(x)=w382:fxp<+,32,16>)
        n169 = Absolute Value(x=w387) -> (abs(x)=w386:fxp<+,32,16>)
        n170 = Divide(x=w386, y=w363) -> (x/y=w359:fxp<+/-,64,33>)
        "# of Points per Line" <- w359
        n171 = Divide(x=w382, y=w368) -> (x/y=w383:fxp<+/-,64,33>)
        n172 = Divide(x=w359, y=w379) -> (x/y=w358:dbl)
        "sec per line" <- w358
        n173 = Add(x=w383, y=fxp<+,16,16> 1.0) -> (x+y=w381:fxp<+/-,64,34>)
        "# of Hor Lines" <- w381
        n174 = Reciprocal(x=w358) -> (1/x=→"line per sec (Hz)":dbl)
        n175 = Multiply(x=w358, y=w381) -> (x*y=→"Total Scan Time (sec)":dbl)
        n176 = Multiply(x=w381, y=w359) -> (x*y=→"# Total Trigger Points":fxp<+/-,64,67>)
        n177 = xnode "Read/Write Control"("FPGA VI Reference In"=w378, "error in"=w365, "XY Reference Loop Period (us)"="XY Reference Time Period (uSec)", "Z Reference Loop Period (us)"="Z Reference Time Period (uSec)", "Scan Geometry"=w354, "X Reference Amplitude (nm)"="X Reference Amplitude (nm)", "Y Reference Amplitude (nm)"="Y Reference Amplitude (nm)", "Z Reference Amplitude (nm)"="Z Reference Amplitude (nm)", "Traj Frequency"=w371, "X Reference DC Offset (nm)"="X Reference DC Offset (nm)", "Y Reference DC Offset (nm)"="Y Reference DC Offset (nm)", "Z Reference DC Offset (nm)"="Z Reference DC Offset (nm)", "Scan type"=w353, "Inner Scan axis"=w355, "Spiral Rotation Direction"=w356, "Radial direction"=w357, "X Start (nm)"=w370, "X End (nm)"=w364, "X Step Size"=w363, "Y Start (nm)"=w362, "Y End (nm)"=w369, "Y Step Size"=w368, "Max radius"=w360, "Spiral Step Size"=w361) -> ("FPGA VI Reference Out"=w376:refnum<k20>, "error out"=w375:errorcluster)
      }
      frame "Update Detector Trigger Info" {
        w459 = 40000000.0  # FPGA clock rate (Hz)
        n178 = case shown="\"EPICS Control\"" w448 {
          tunnel: ["DT Frequency (Hz)" w471] -> w460
          tunnel: ["DT duty cycle (%)" w470] -> w455
          frame "Local Control", Default {
          }
          frame "EPICS Control" {
            n179 = shared-variable "RT CompactRIO Target\\RT_EPICS_Shared_Variables.lvlib\\2iddVELO:VP:Trig_DutyCycle_Per"() -> (w470:dbl)  [unwired: 1 in, 1 out]
            "2iddVELO:VP:Trig_DutyCycle_Per" <- w470
            n180 = shared-variable "RT CompactRIO Target\\RT_EPICS_Shared_Variables.lvlib\\2iddVELO:VP:Trigger_Freq_Hz"() -> (w471:dbl)  [unwired: 1 in, 1 out]
          }
        }
        "Trigger Frequency (Hz)" <- w460
        "Trigger Duty Cycle (%)" <- w455
        n181 = call <vilib>:"Normalize Signal Generation Parameters.vi"("frequency (Hz)"=w460, "FPGA clock rate (Hz)"=w459, "phase offset (deg)"="DT phase offset (deg)", "duty cycle (%)"=w455, "error in (no error)"=w446) -> ("frequency (periods/tick)"=w458:fxp<+,32,0>, "phase offset (periods)"=w457:fxp<+,32,0>, "duty cycle (periods)"=w456:fxp<+,32,0>, "error out"=w445:errorcluster)  [unwired: 5 in, 2 out]
        "DT Frequency (periods/tick)" <- w458
        "DT Phase Offset (periods)" <- w457
        "DT Duty Cycle (periods)" <- w456
        n182 = xnode "Read/Write Control"("FPGA VI Reference In"=w454, "error in"=w445, "Trigger Generation Time Period (uSec)"="Trigger Generation Time Period (uSec)", "Detector Trigger Lower Limit (V)"="Detector Trigger Lower Limit (V)", "Detector Trigger Upper Limit (V)"="Detector Trigger Upper Limit (V)", "DT Reference Amplitude (V)"="DT Reference Amplitude (V)", "DT Reference DC Offset (V)"="DT Reference DC Offset (V)", "Det Frequency"=w458, "DT Phase Offset (periods)"=w457, "DT Reset"="DT Reset", "DT Duty Cycle (periods)"=w456) -> ("FPGA VI Reference Out"=w452:refnum<k20>, "error out"=w451:errorcluster)
      }
      frame "Update Datalog Info" {
        n183 = xnode "Read/Write Control"("FPGA VI Reference In"=w482, "error in"=w481, "FIFO Loop Period (us)"="Datalog Time Period (uSec)", "Datalog Cases"="Datalog Cases", "Timeout FPGA FIFO1"="Timeout FPGA FIFO1", "Data Save Trigger Source"="Data Save Trigger Source") -> ("FPGA VI Reference Out"=w479:refnum<k20>, "error out"=w478:errorcluster)
      }
      frame "Check FPGA Status" {
        n184 = xnode "Read/Write Control"("FPGA VI Reference In"=w496, "error in"=w495) -> ("FPGA VI Reference Out"=w494:refnum<k20>, "error out"=w493:errorcluster, "FPGA error monitor"=w499:errorcluster, "End Run Error"=w498:errorcluster, "FIFO Timed Out?"=→"FIFO Timed Out?":bool, "Stop Scan"=w488:bool, "FIFO Timed Out"=w489:bool)
        "FPGA end run error" <- w498
        "Stop Run" <- w488
        "FIFO Timed Out" <- w489
        n185 = case shown="True" w488 {
          tunnel: [errorcluster {"status"=FALSE, "code"=0, "source"=""} ("error constant") errorcluster {"status"=TRUE, "code"=7002, "source"="FPGA stop case encountered"} ("error constant")] -> w486
          frame False {
          }
          frame True {
          }
        }
        n186 = case shown="True" w489 {
          tunnel: [errorcluster {"status"=FALSE, "code"=0, "source"=""} ("error constant") errorcluster {"status"=TRUE, "code"=7001, "source"="FPGA FIFO timed out"} ("error constant")] -> w487
          frame False {
          }
          frame True {
          }
        }
        n187 = Merge Errors(w493, w499, w498, w486, w487) -> (w485:errorcluster)
      }
      frame "Pre-Scan" {
        n188 = flat-sequence {
          tunnel: w518 -> [w526]
          tunnel: w517 -> [w525]
          tunnel: [w522] -> w516
          tunnel: [w521] -> w514
          tunnel: w516 -> [w531]
          tunnel: [w531] -> w515
          tunnel: w514 -> [w530]
          tunnel: [w530] -> w513
          tunnel: w515 -> [w535]
          tunnel: w513 -> [w534]
          tunnel: [w533] -> w512
          tunnel: [w532] -> w511
          tunnel: w512 -> [w543]
          tunnel: w511 -> [w542]
          tunnel: [w539] -> w506
          tunnel: [w538] -> w505
          tunnel: [w545] -> w509
          tunnel: [w547] -> w510
          tunnel: w506 -> [w548]
          tunnel: w505 -> [w546]
          tunnel: w504 -> [w544]
          frame #0 {
            w523 = TRUE
            n189 = xnode "Read/Write Control"("FPGA VI Reference In"=w526, "error in"=w525, "Reset Optics X"=w523, "Reset Optics Y"=w523, "Reset Optics Z"=w523, "Reset Sample X"=w523, "Reset Sample Y"=w523, "Reset Sample Z"=w523, "System Loop Type"=enum16{"Open Loop", "Closed Loop"}."Open Loop", "New FPGA command"=TRUE, "FPGA command"=enum16{"Start Scan", "Shutdown"}."Start Scan", "Data Save Flag"=enum16{"Skip Data", "Save Data"}."Skip Data") -> ("FPGA VI Reference Out"=w522:refnum<k20>, "error out"=w521:errorcluster)
          }
          frame #1 {
            n190 = Wait (ms)(milliseconds to wait="Pre-Scan pause (ms)") -> ()  [unwired: 1 out]
          }
          frame #2 {
            n191 = xnode ("Read/Write Control")("FPGA VI Reference In"=w535, "error in"=w534, "Stop Scan"=TRUE ("stop case")) -> ("FPGA VI Reference Out"=w533:refnum<k20>, "error out"=w532:errorcluster)
          }
          frame #3 {
            w540 = FALSE ("Reset Optics X")
            n192 = local read "System Loop Type"() -> (w541:enum16{"Open Loop", "Closed Loop"})
            n193 = xnode "Read/Write Control"("FPGA VI Reference In"=w543, "error in"=w542, "Reset Optics X"=w540, "Reset Optics Y"=w540, "Reset Optics Z"=w540, "Reset Sample X"=w540, "Reset Sample Y"=w540, "Reset Sample Z"=w540, "System Loop Type"=w541, "Data Save Flag"="Data Save Flag") -> ("FPGA VI Reference Out"=w539:refnum<k20>, "error out"=w538:errorcluster)
          }
          frame #4 {
            n194 = case shown="\"Fly\", Default" w544 {
              tunnel: w548 -> [w554 w558]
              tunnel: [w550 w558] -> w547
              tunnel: w546 -> [w553 w557]
              tunnel: [w549 w557] -> w545
              frame "Fly", Default {
                n195 = xnode ("Invoke Method")("FPGA VI Reference In"=w554, "error in"=w553, "Requested Depth"="Requested Depth") -> ("FPGA VI Reference Out"=w552:refnum<k20>, "error out"=w551:errorcluster, "Actual Depth"=→"Actual Depth":u32)
                n196 = xnode "Invoke Method"("FPGA VI Reference In"=w552, "error in"=w551) -> ("FPGA VI Reference Out"=w550:refnum<k20>, "error out"=w549:errorcluster)
              }
              frame "Step" {
              }
            }
          }
        }
      }
      frame "Start Scan" {
        n197 = xnode "Read/Write Control"("FPGA VI Reference In"=w572, "error in"=w571, "Scan type"=w569) -> ("FPGA VI Reference Out"=w561:refnum<k20>, "error out"=w570:errorcluster)
        n198 = case shown="\"Fly\", Default" w569 {
          tunnel: [w578 w586] -> w562
          tunnel: w570 -> [w577 w586]
          frame "Fly", Default {
            n199 = shared-variable ".\\Interloop communication.lvlib\\Base Filename"() -> (w579:string)  [unwired: 1 in, 1 out]
            n200 = String To Path(string="cRIO data dir") -> (path=w580:path)
            "cRIO path" <- w580
            n201 = call "Data_Write.vi"("Destination dir"=w580, "error initialize"=w577, "Base name"=w579, "Command List"=Data_Write_Control."Initialize") -> ("error out"=w578:errorcluster, "Path"=w584:path)  [unwired: 4 in]
            n202 = Strip Path(path=w584) -> (stripped path=→"Output path":path, name=→"Output filename":string)
          }
          frame "Step" {
          }
        }
        n203 = xnode "Read/Write Control"("FPGA VI Reference In"=w561, "error in"=w562) -> ("FPGA VI Reference Out"=w560:refnum<k20>, "error out"=w563:errorcluster, "Trajectory Complete"=w559:bool)
        n204 = shared-variable "RT CompactRIO Target\\RT_EPICS_Shared_Variables.lvlib\\2iddVELO:VP:Scanning"(TRUE ("2iddVELO:VP:Scanning")) -> ()  [unwired: 1 in, 1 out]
        n205 = local write "Trajectory Completed"(w559) -> ()
        n206 = xnode "Read/Write Control"("FPGA VI Reference In"=w560, "error in"=w563, "New FPGA command"=TRUE, "FPGA command"=enum16{"Start Scan", "Shutdown"}."Start Scan") -> ("FPGA VI Reference Out"=w567:refnum<k20>, "error out"=w566:errorcluster)
      }
      frame "Step Scanning" {
        n207 = case shown="\"EPICS Control\"" w588 {
          tunnel: [w603 w605] -> w590
          tunnel: [w604 w608] -> w591
          tunnel: [w602 w606] -> w589
          frame "Local Control", Default {
            n208 = local read "X Reference Amplitude (nm)"() -> (w602:fxp<+/-,40,17>)
            n209 = local read "Y Reference Amplitude (nm)"() -> (w603:fxp<+/-,40,17>)
            n210 = local read "Z Reference Amplitude (nm)"() -> (w604:fxp<+/-,40,17>)
          }
          frame "EPICS Control" {
            w607 = fxp<+/-,40,17> 0.0 ("Z Reference Amplitude (nm)")
            n211 = shared-variable "RT CompactRIO Target\\RT_EPICS_Shared_Variables.lvlib\\2iddVELO:LabView:ZPZ_Command"() -> (w609:dbl)  [unwired: 1 in, 1 out]
            n212 = shared-variable "RT CompactRIO Target\\RT_EPICS_Shared_Variables.lvlib\\2iddVELO:LabView:ZPY_Command"() -> (w610:dbl)  [unwired: 1 in, 1 out]
            n213 = shared-variable "RT CompactRIO Target\\RT_EPICS_Shared_Variables.lvlib\\2iddVELO:LabView:ZPX_Command"() -> (w611:dbl)  [unwired: 1 in, 1 out]
            n214 = To Fixed-Point(fixed-point type=w607, number=w611) -> (fixed-point=w606:fxp<+/-,40,17>)
            n215 = To Fixed-Point(fixed-point type=w607, number=w610) -> (fixed-point=w605:fxp<+/-,40,17>)
            n216 = To Fixed-Point(fixed-point type=w607, number=w609) -> (fixed-point=w608:fxp<+/-,40,17>)
            n217 = local write "X Reference Amplitude (nm)"(w606) -> ()
            n218 = local write "Y Reference Amplitude (nm)"(w605) -> ()
            n219 = local write "Z Reference Amplitude (nm)"(w608) -> ()
          }
        }
        n220 = xnode "Read/Write Control"("FPGA VI Reference In"=w595, "error in"=w594, "X Reference Amplitude (nm)"=w589, "Y Reference Amplitude (nm)"=w590, "Z Reference Amplitude (nm)"=w591) -> ("FPGA VI Reference Out"=w593:refnum<k20>, "error out"=w592:errorcluster)
        n221 = Insert Into Array(array=w601, index=0, new element=State_Enum."Step Scanning" ("new element/subarray")) -> (w600:T10[])
      }
      frame "Fly Scanning" {
        n222 = xnode "Read/Write Control"("FPGA VI Reference In"=w639, "error in"=w620) -> ("FPGA VI Reference Out"=w634:refnum<k20>, "error out"=w633:errorcluster, "FPGA state"=w629:T9)
        n223 = Equal?(x=T9."Wait", y=w629) -> (x = y?=w626:bool)
        n224 = xnode "Invoke Method"("FPGA VI Reference In"=w634, "error in"=w633, "Number of Elements"=u32 0, "Timeout (ms)"=100) -> ("FPGA VI Reference Out"=w631:refnum<k20>, "error out"=w632:errorcluster, "Elements Remaining"=w615:u32)  [unwired: 1 out]
        "Elements Available in FIFO" <- w615
        n225 = Equal?(x=u32 0, y=w615) -> (x = y?=w627:bool)
        n226 = Compound Arithmetic op=AND(w613, w626, w627) -> (w625:bool)
        n227 = xnode ("Invoke Method")("FPGA VI Reference In"=w631, "error in"=w632, "Number of Elements"=w615, "Timeout (ms)"="FIFO Timeout (ms)") -> ("FPGA VI Reference Out"=w617:refnum<k20>, "error out"=w638:errorcluster, "Data"=w621:fxp<+/-,40,32>[], "Elements Remaining"=→"Elements Remaining" →"Elements Remaining in FIFO":u32)
        "Data" <- w621
        n228 = Enqueue Element(queue=w618, element=w621, error in (no error)=w620) -> (error out=w619:errorcluster)  [unwired: 1 in, 2 out]
        n229 = case shown="False" w625 {
          tunnel: w624 -> [w644 w645]
          tunnel: [w642 w645] -> w623
          frame False {
            # "Either FIFO not empty or FPGA not \ndone running -- repeat scanning state"
            n230 = Insert Into Array(array=w644, index=0, new element=State_Enum."Fly Scanning" ("new element/subarray")) -> (w642:T10[])
          }
          frame True {
            # "FIFO empty, FPGA done running \n-- moving onto next state"
          }
        }
        n231 = Merge Errors(w638, w619) -> (w637:errorcluster)
      }
      frame "End Scan" {
        n232 = case shown="\"Fly\", Default" w651 {
          tunnel: w656 -> [w663 w664]
          tunnel: [w662 w664] -> w655
          tunnel: w654 -> [w661 w665]
          tunnel: [w660 w665] -> w653
          frame "Fly", Default {
            n233 = xnode "Invoke Method"("FPGA VI Reference In"=w663, "error in"=w661) -> ("FPGA VI Reference Out"=w662:refnum<k20>, "error out"=w660:errorcluster)
          }
          frame "Step" {
          }
        }
        n234 = xnode "Read/Write Control"("FPGA VI Reference In"=w655, "error in"=w653, "Stop Scan"=TRUE ("New FPGA command")) -> ("FPGA VI Reference Out"=w650:refnum<k20>, "error out"=w648:errorcluster)
        n235 = shared-variable "RT CompactRIO Target\\RT_EPICS_Shared_Variables.lvlib\\2iddVELO:VP:Scanning"(FALSE ("2iddVELO:VP:Fly_Scanning"), error in=w648) -> (error out=w647:errorcluster)
      }
      frame "Close File" {
        n236 = local read "Queue is empty"() -> (w667:bool)
        n237 = case shown="True" w667 {
          tunnel: [w679 w683] -> w674
          tunnel: w670 -> [w679 w682]
          tunnel: w672 -> [w676 w680]
          tunnel: [w675 w680] -> w673
          frame False {
            # "Queue is not empty, so file is still be written to"
            n238 = Insert Into Array(array=w676, index=0, new element=State_Enum."Close File" ("new element/subarray")) -> (w675:T10[])
          }
          frame True {
            n239 = call "Data_Write.vi"("error initialize"=w682, "Command List"=Data_Write_Control."Close") -> ("error out"=w681:errorcluster)  [unwired: 6 in, 1 out]
            n240 = case shown="No Error" w681 {
              tunnel: w681 -> [w690 w691]
              tunnel: [w689 w691] -> w683
              frame No Error {
                n241 = local read "Output filename"() -> (w685:string)
                n242 = local read "Output path"() -> (w686:path)
                n243 = Path To String(path=w686) -> (string=w688:string)
                n244 = shared-variable "RT CompactRIO Target\\RT_EPICS_Shared_Variables.lvlib\\2iddVELO:VP:Last_Filename"(w685, error in=w690) -> (error out=w687:errorcluster)
                n245 = shared-variable "RT CompactRIO Target\\RT_EPICS_Shared_Variables.lvlib\\2iddVELO:VP:cRIO_Dir"(w688, error in=w687) -> (error out=w689:errorcluster)
              }
              frame Error {
              }
            }
          }
        }
      }
      frame "Restart FPGA" {
        n246 = call <vilib>:"Clear Errors.vi"("error in (no error)"=w698) -> ("error out"=w699:errorcluster)  [unwired: 5 in, 1 out]
        n247 = xnode "Invoke Method"("FPGA VI Reference In"=w704, "error in"=w699) -> ("FPGA VI Reference Out"=w703:refnum<k20>, "error out"=w702:errorcluster)
        n248 = xnode "Read/Write Control"("FPGA VI Reference In"=w703, "error in"=w702, "Stop Scan"=TRUE ("stop case")) -> ("FPGA VI Reference Out"=w697:refnum<k20>, "error out"=w696:errorcluster)
        n249 = xnode "Invoke Method"("FPGA VI Reference In"=w697, "error in"=w696) -> ("FPGA VI Reference Out"=w695:refnum<k20>, "error out"=w694:errorcluster)
      }
      frame "Stop FPGA" {
        w713 = T10[] [enum."Stop FPGA"] items=["Initialization", "Import Controller coeffs", "Update Controller Info", "Wait", "Update Reference Info", "Update Detector Trigger Info", "Update Datalog Info", "Check FPGA Status", "Initialize FIFO", "Pre-Scan", "Start Scan", "Step Scanning", "Fly Scanning", "End Scan", "Close File", "Restart FPGA", "Stop FPGA"] ("Reduced Array of States")
        w712 = TRUE ("stop case")
        n250 = xnode "Invoke Method"("FPGA VI Reference In"=w720, "error in"=w719) -> ("FPGA VI Reference Out"=w718:refnum<k20>, "error out"=w717:errorcluster)
        n251 = xnode "Read/Write Control"("FPGA VI Reference In"=w718, "error in"=w717, "Stop Scan"=w712, "New FPGA command"=w712, "FPGA command"=enum16{"Start Scan", "Shutdown"}."Shutdown") -> ("FPGA VI Reference Out"=w716:refnum<k20>, "error out"=w709:errorcluster)
        n252 = xnode "Invoke Method"("FPGA VI Reference In"=w716, "error in"=w709) -> ("FPGA VI Reference Out"=w710:refnum<k20>, "error out"=w708:errorcluster)
        n253 = xnode "Close FPGA VI Reference"("FPGA VI Reference In"=w710, "error in"=w708) -> ("error out"=w715:errorcluster)
      }
    }
    "Main Loop error" <- w188
    n254 = shared-variable ".\\Interloop communication.lvlib\\Main Loop Error"(w188) -> ()  [unwired: 1 in, 1 out]
    n255 = node-c288(w193) -> ()  [unwired: 1 out]
    n256 = call "State Control.vi"("Stop"=FALSE, "Array of States"=w198, "Error Input"=w188) -> ("Next State"=w190:T10, "Reduced Array of States"=w194:T10[])  [unwired: 5 in]
    "RT Main Loop State" <- w184
    "Main Loop Iterations" <- w196
    "Reduced Array of States" <- w195
  }
  n257 = while {
    tunnel: w3 -> [w743]
    shift-right: [w734] -> _
    shift-left: w2 -> [w742]
    shift-right: [w727] -> _
    shift-left: _ -> [w726]
    i -> [w733]
    stop <- w735 stop-if-true
    n258 = Get Queue Status(queue=w743, error in (no error)=w742) -> (queue out=w740:refnum<queue>, error out=w741:errorcluster, # elements in queue=w738:i32)  [unwired: 1 in, 5 out]
    n259 = Greater Than 0?(x=w738) -> (x > 0?=w739:bool)
    n260 = case shown="True" w739 {
      tunnel: w741 -> [w750 w780]
      tunnel: w740 -> [_ w779]
      tunnel: [w750 w777] -> w734
      tunnel: [TRUE FALSE] -> w732
      tunnel: [w744 w765] -> w727
      tunnel: w726 -> [w746 w764]
      frame False {
        n261 = local read "RT Main Loop State"() -> (w749:T10)
        n262 = Equal?(x=w749, y=State_Enum."Fly Scanning") -> (x = y?=w747:bool)
        n263 = Select(t=w746, s=w747, f=fxp<+/-,58,25>[] []) -> (s? t:f=w744:fxp<+/-,58,25>[])
      }
      frame True {
        w772 = 0.0  # t0
        w784 = "%8f"  # format string
        w785 = ","  # delimiter (Tab)
        n264 = local read "Trigger Frequency (Hz)"() -> (w774:dbl)
        "Data Read Rate (Hz)" <- w774
        n265 = Dequeue Element(queue=w779, error in (no error)=w780) -> (element=w755:fxp<+/-,58,25>[], error out=w778:errorcluster)  [unwired: 1 in, 2 out]
        n266 = Array Size(array=w764) -> (size(s)=w763:i32)
        n267 = Insert Into Array(array=w764, index=w763, new element=w755) -> (w765:fxp<+/-,58,25>[])
        n268 = Decimate 1D Array(w755) -> (w760:fxp<+/-,58,25>[], w759:fxp<+/-,58,25>[], w758:fxp<+/-,58,25>[], w757:fxp<+/-,58,25>[], w756:fxp<+/-,58,25>[])
        n269 = Decimate 1D Array(w765) -> (w787:fxp<+/-,58,25>[], w788:fxp<+/-,58,25>[], w789:fxp<+/-,58,25>[], w790:fxp<+/-,58,25>[], w782:fxp<+/-,58,25>[])
        n270 = Build Array(w760, w759, w758, w757, w756) -> (w754:fxp<+/-,58,25>[][])
        n271 = Build Array(w787, w788, w789, w790, w782) -> (w781:fxp<+/-,58,25>[][])
        n272 = To Double Precision Float(number=w754) -> (double precision float=w753:dbl[][])
        n273 = Reciprocal(x=w774) -> (1/x=w771:dbl)
        "Data Read Period (sec)" <- w771
        n274 = To Double Precision Float(number=w781) -> (double precision float=w752:dbl[][])
        n275 = Transpose 2D Array(2D array=w753) -> (transposed array=w776:dbl[][])
        n276 = Bundle("t0"=w772, w771, w752) -> (→"Reference and Actual positions":cluster{"t0":dbl, dbl, dbl[][]})  [unwired: 1 in]
        n277 = To Double Precision Float(number=w787) -> (double precision float=w769:dbl[])
        n278 = To Double Precision Float(number=w788) -> (double precision float=w768:dbl[])
        n279 = To Double Precision Float(number=w789) -> (double precision float=w767:dbl[])
        n280 = To Double Precision Float(number=w790) -> (double precision float=w766:dbl[])
        n281 = Bundle(w767, w766) -> (w761:cluster{dbl[], dbl[]})  [unwired: 1 in]
        n282 = Bundle(w769, w768) -> (w770:cluster{dbl[], dbl[]})  [unwired: 1 in]
        n283 = Array To Spreadsheet String(delimiter (Tab)=w785, array=w776, 3:w784) -> (spreadsheet string=w786:string)
        n284 = Build Array(w770, w761) -> (→"XY Ref":cluster{dbl[], dbl[]}[])
        n285 = call "Data_Write.vi"("error initialize"=w778, "Data"=w786, "Command List"=Data_Write_Control."Write") -> ("error out"=w777:errorcluster)  [unwired: 5 in, 1 out]
      }
    }
    "File Writer loop error" <- w734
    "Queue is empty" <- w732
    n286 = local read "Stop System (Careful!!)"() -> (w736:bool)
    n287 = Equal To 0?(x=w738) -> (x = 0?=w737:bool)
    n288 = And(x=w736, y=w737) -> (x .and. y?=w735:bool)
    n289 = local read "Fly scan loop dt"() -> (w729:i64)
    n290 = Divide(x=w729, y=i64 2) -> (x/y=w730:dbl)
    n291 = To Unsigned Long Integer(number=w730) -> (unsigned 32bit integer=w728:u32)
    n292 = Wait Until Next ms Multiple(millisecond multiple=w728) -> ()  [unwired: 1 out]
    "File writer loop iterations" <- w733
  }
  n293 = while {
    shift-right: [w804] -> _
    shift-left: TRUE -> [w805]
    i -> [w793]
    stop <- w797 stop-if-true
    # "Heartbeat Loop"
    n294 = shared-variable ".\\Interloop communication.lvlib\\EPICS command error"() -> (w791:errorcluster)  [unwired: 1 in, 1 out]
    n295 = shared-variable ".\\Interloop communication.lvlib\\Command Loop Error"() -> (w799:errorcluster)  [unwired: 1 in, 1 out]
    n296 = shared-variable ".\\Interloop communication.lvlib\\FPGA startup error"() -> (w796:errorcluster)  [unwired: 1 in, 1 out]
    n297 = Not(x=w805) -> (.not. x?=w804:bool)
    "Heartbeat" <- w804
    n298 = shared-variable ".\\Interloop communication.lvlib\\Readback Loop Error"() -> (w798:errorcluster)  [unwired: 1 in, 1 out]
    n299 = shared-variable ".\\Interloop communication.lvlib\\Main Loop Error"() -> (w803:errorcluster)  [unwired: 1 in, 1 out]
    n300 = call <vilib>:"RT LEDs.vi"("State"=3, "LED Num"=0) -> ("error out"=w792:errorcluster)  [unwired: 4 in, 1 out]
    n301 = Merge Errors(w792, w791, w799, w796, w803, w798) -> (w800:errorcluster)
    n302 = case shown="No Error" w800 {
      selector: w800 -> [w806 w808]
      tunnel: [u32 500 ("millisecond multiple") u32 100 ("millisecond multiple")] -> w802
      tunnel: [w806 w808] -> w801
      frame No Error {
      }
      frame Error {
      }
    }
    "RT error" <- w801
    n303 = local read "Stop System (Careful!!)"() -> (w797:bool)
    n304 = Wait Until Next ms Multiple(millisecond multiple=w802) -> ()  [unwired: 1 out]
    "Heartbeat Loop Iterations" <- w793
  }
  n305 = while {
    stop <- w846 stop-if-true
    n306 = shared-variable "RT CompactRIO Target\\RT_EPICS_Shared_Variables.lvlib\\2iddVELO:VP:Radial_Direction"() -> (w819:string, error out=w821:errorcluster)  [unwired: 1 in]
    "2iddVELO:VP:Radial_Direction" <- w819
    n307 = shared-variable "RT CompactRIO Target\\RT_EPICS_Shared_Variables.lvlib\\2iddVELO:VP:Rotation_Direction"() -> (w826:string, error out=w825:errorcluster)  [unwired: 1 in]
    "2iddVELO:VP:Rotation_Direction" <- w826
    n308 = shared-variable "RT CompactRIO Target\\RT_EPICS_Shared_Variables.lvlib\\2iddVELO:VP:Inner_Scan_Axis"() -> (w812:string, error out=w820:errorcluster)  [unwired: 1 in]
    "2iddVELO:VP:Inner_Scan_Axis" <- w812
    n309 = shared-variable "RT CompactRIO Target\\RT_EPICS_Shared_Variables.lvlib\\2iddVELO:VP:Controller_Type"() -> (w844:string, error out=w837:errorcluster)  [unwired: 1 in]
    "2iddVELO:VP:Controller_Type" <- w844
    n310 = shared-variable "RT CompactRIO Target\\RT_EPICS_Shared_Variables.lvlib\\2iddVELO:VP:Scan_Trajectory"() -> (w831:string, error out=w829:errorcluster)  [unwired: 1 in]
    "2iddVELO:VP:Scan_Trajectory" <- w831
    n311 = shared-variable "RT CompactRIO Target\\RT_EPICS_Shared_Variables.lvlib\\2iddVELO:VP:cRIO_Command"() -> (w843:string, error out=w839:errorcluster)  [unwired: 1 in]
    "2iddVELO:VP:cRIO_Command" <- w843
    n312 = shared-variable "RT CompactRIO Target\\RT_EPICS_Shared_Variables.lvlib\\2iddVELO:VP:Scan_Type"() -> (w842:string, error out=w835:errorcluster)  [unwired: 1 in]
    "2iddVELO:VP:Scan_Type" <- w842
    n313 = Scan From String(input string=w819, error in=w821, default 1=enum16{"Outward", "Inward"}."Outward" ("EPICS radial direction 2")) -> (error out=w822:errorcluster, output 1=→"EPICS radial direction":enum16{"Outward", "Inward"})  [unwired: 2 in, 2 out]
    n314 = Scan From String(input string=w812, error in=w820, default 1=enum16{"X", "Y"}."X" ("EPICS Inner axis 2")) -> (error out=w823:errorcluster, output 1=→"EPICS Inner axis":enum16{"X", "Y"})  [unwired: 2 in, 2 out]
    n315 = Scan From String(input string=w826, error in=w825, default 1=enum16{"Clockwise", "Anti-clockwise"}."Anti-clockwise" ("Rotation Direction 2")) -> (error out=w824:errorcluster, output 1=→"EPICS rotation direction":enum16{"Clockwise", "Anti-clockwise"})  [unwired: 2 in, 2 out]
    n316 = Scan From String(input string=w843, error in=w839, default 1=EPICS_Command_Control."Start Scan" ("default value 1")) -> (error out=w838:errorcluster, output 1=→"EPICS cRIO Command":T5)  [unwired: 2 in, 2 out]
    n317 = Scan From String(input string=w831, error in=w829, default 1=T3."Archimedes Spiral" ("Scan Geometry")) -> (error out=w828:errorcluster, output 1=→"EPICS Scan Trajectory":T3)  [unwired: 2 in, 2 out]
    n318 = Scan From String(input string=w844, error in=w837, default 1=Controller_Type."H-infinity" ("Controller Type")) -> (error out=w836:errorcluster, output 1=→"EPICS Controller Type":T2)  [unwired: 2 in, 2 out]
    n319 = Scan From String(input string=w842, error in=w835, default 1=enum16{"Fly", "Step"}."Fly" ("Scan type 2")) -> (error out=w834:errorcluster, output 1=→"EPICS Scan Type":enum16{"Fly", "Step"})  [unwired: 2 in, 2 out]
    n320 = local read "Stop System (Careful!!)"() -> (w846:bool)
    n321 = Merge Errors(w822, w823, w824, w828, w838, w836, w834) -> (w833:errorcluster)
    "EPICS command error" <- w833
    n322 = shared-variable ".\\Interloop communication.lvlib\\EPICS command error"(w833) -> ()  [unwired: 1 in, 1 out]
    n323 = Wait Until Next ms Multiple(millisecond multiple=u32 100) -> ()  [unwired: 1 out]
  }
  n324 = node-c288(w12) -> (→"Timed Loop (end error)":errorcluster, →"Iteration Duration RT Timed-Loop":i64)
  n325 = Release Queue(queue=w3, error in (no error)=w4) -> ()  [unwired: 1 in, 3 out]
